vi "Main 手動測試.vi"() -> ()   [LabVIEW 2015]
uses:
  <vilib>/Utility/miscctls.llb/LVPointTypeDef.ctl
  2.0_Function/Function_VISA/Control/Control_Motion Action.ctl
  2.0_Function/Function_VISA/Control/Control_Axis Number.ctl
  <vilib>/Instr/_visa.llb/Select Event Type.ctl
panel:
  out "急停":bool
  out "DI":bool[][](array[boolean])
  in  "Time":u32=15000
  in  "儲存日檢位":path=path "D:/全域高斯機 參數/Daily Check"
  in  "儲存每日檢測位":bool
  out "量測值(T)":dbl format="%.1f"
  in  "單步角度(degree)":dbl=1.0 format="%#_13g"
  in  "確認離開":bool
  in  "單步距離(mm)":dbl=1.0 format="%#_13g"
  in  "-Rotation":bool
  in  "匯入硬體參數":path=path "D:/全域高斯機 參數/Paremeter"
  in  "目前位置":T1
  in  "軸參數":T2={"Name"="7", "VISA In"="COM2", "R"=0.0, "Y"=0.0, "Z"=0.0, "θ"=0.0, "最大值"=2.0, "最小值"=0.0, "VISA Data"={"Baud rate"=115200, "Data bits"=8, "Parity"=enum."Even", "Stop bits"=10, "Flow control"=0}, "Paremeter"={"Scan speed"=4, "Power"=2, "Angle"=0.0, "X"=3000, "X"=30000, "Xc"=30000}, "DAQ Paremeter"={"Task In"="CalibrationTest", "Physical Channels"="Dev1/ai0", "Max Value"=10.0, "Min Value"=-10.0, "Rate"=5.0}} {"DAQ Paremeter"."Rate" format="%0.2f"; "DAQ Paremeter"."Min Value" format="%0.2f"; "DAQ Paremeter"."Max Value" format="%0.2f"; "VISA Data"."Stop bits" items=["1.0"=10, "1.5"=15, "2.0"=20]; "VISA Data"."Flow control" items=["None", "XON/XOFF", "RTS/CTS", "XON/XOFF & RTS/CTS", "DTR/DSR", "XON/XOFF & DTR/DSR"]; "VISA Data"."Data bits" min=5 max=8 step=1; "Paremeter"."Power" items=["Abs"=2, "Rel"=3]; "Paremeter"."Scan speed" items=["X"=1, "Y"=2, "Z"=3, "Rotation"=4]}
  out "手動測試-Action":T5
  in  "+Z":bool
  in  "-Z":bool
  in  "All Home":bool
  in  "All Servo ON/off":bool
  in  "Rotation":bool
  in  "+X":bool
  in  "-X":bool
  in  "-Y":bool
  in  "+Y":bool
  in  "離開":bool
  # "手動測試"
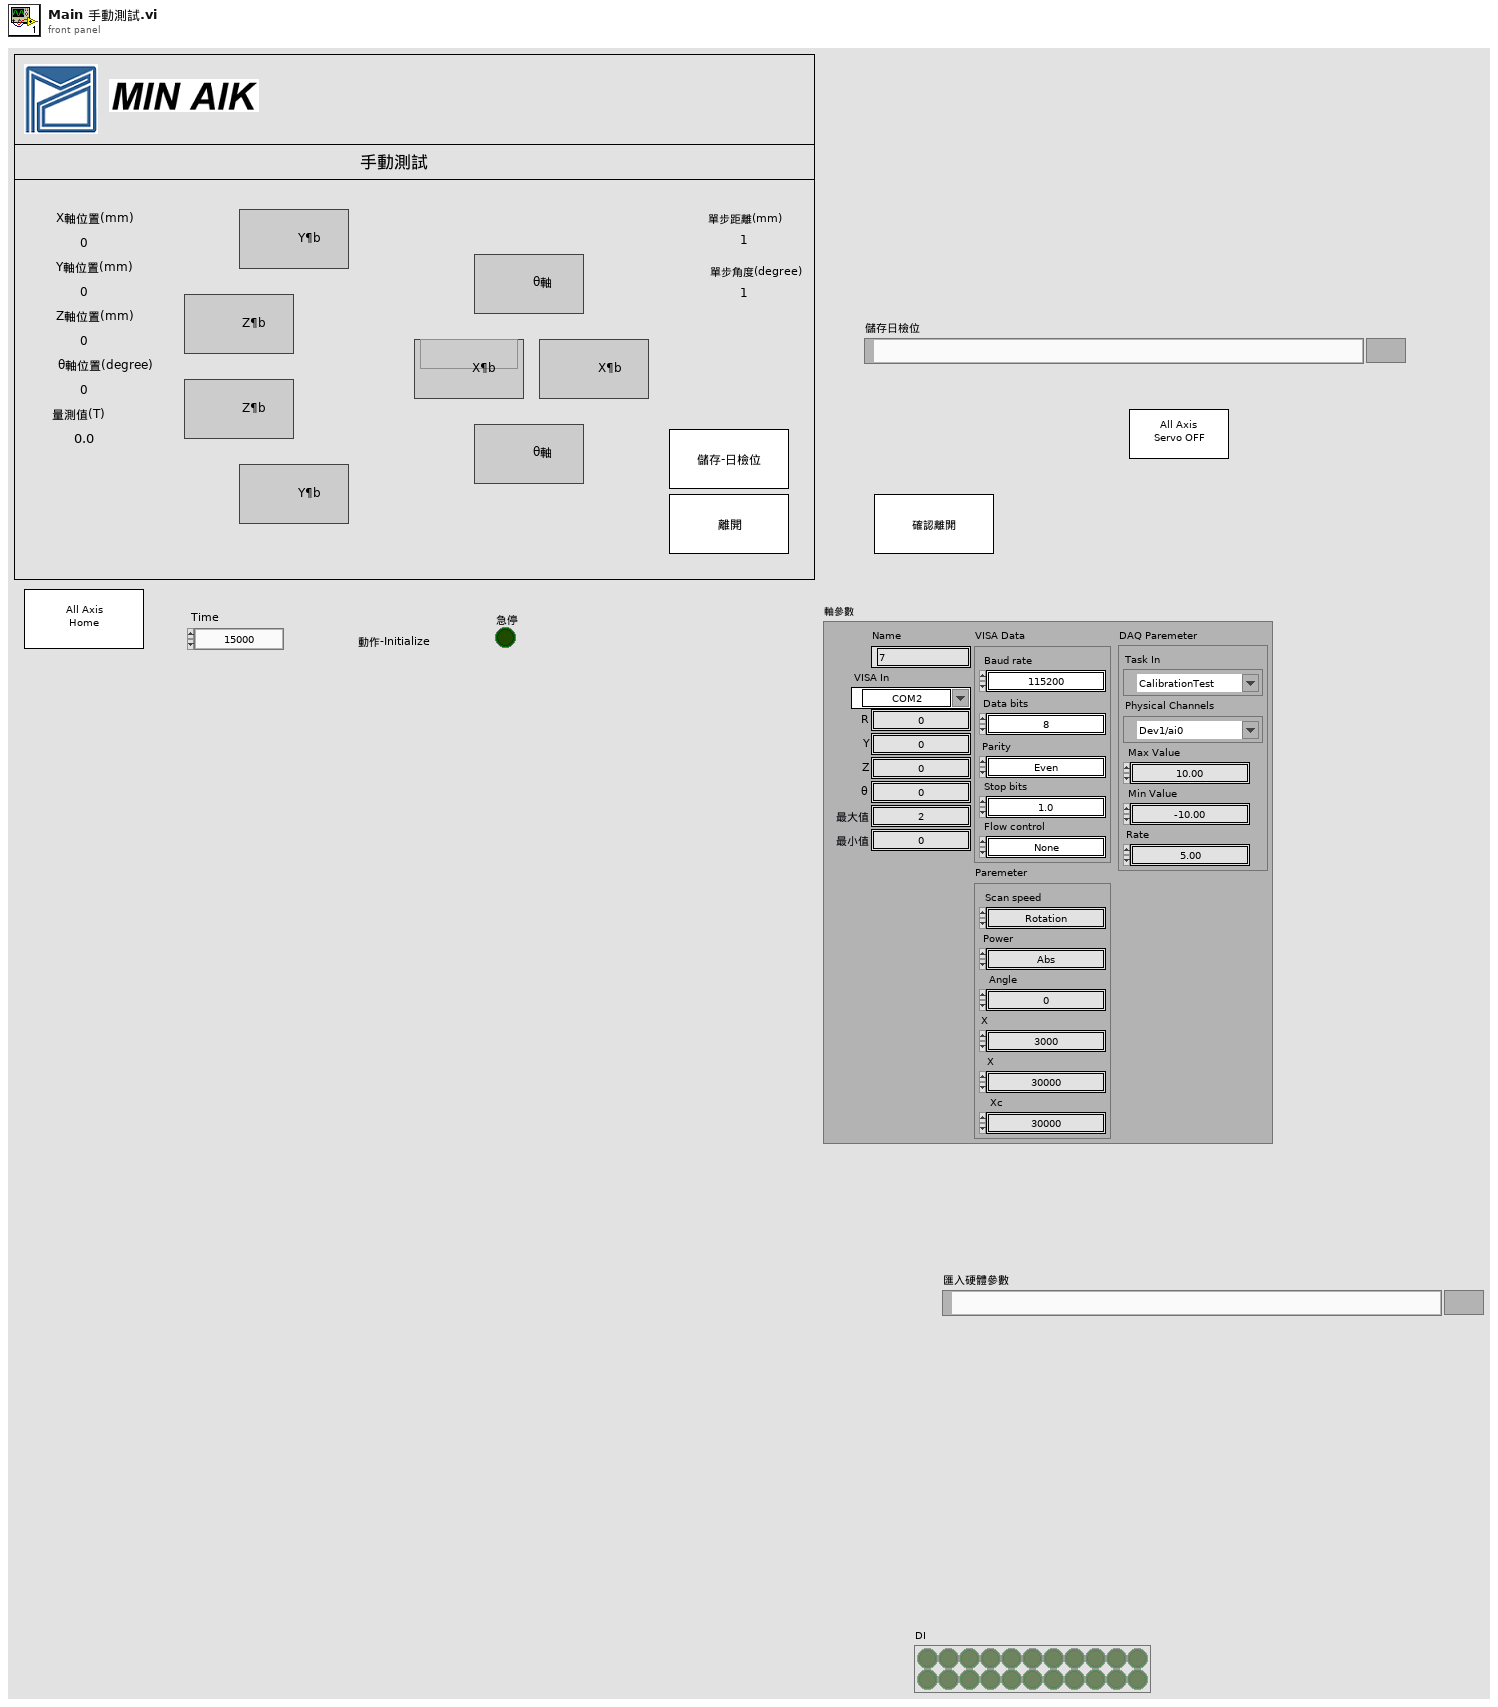
[diagram p1: front panel]
types:
  T1 = cluster{"X軸位置(mm)":dbl, "Y軸位置(mm)":dbl, "Z軸位置(mm)":dbl, "θ軸位置(degree)":dbl}
  T2 = typedef "Control_軸參數.ctl" = cluster{"Name":string, "VISA In":refnum<visa-resource-name>, "R":dbl, "Y":dbl, "Z":dbl, "θ":dbl, "最大值":dbl, "最小值":dbl, "VISA Data":cluster{"Baud rate":u32, "Data bits":u16, "Parity":enum16{"None", "Odd", "Even", "Mark", "Space"}, "Stop bits":u16, "Flow control":u16}, "Paremeter":T3, "DAQ Paremeter":cluster{"Task In":refnum<k21>, "Physical Channels":tag, "Max Value":dbl, "Min Value":dbl, "Rate":dbl}}
  T3 = typedef "Control_手動測試_軸參數.ctl" = cluster{"Scan speed":T4, "Power":u16, "Angle":dbl, "X":i32, "X":i32, "Xc":i32}
  T4 = typedef "Control_Axis Number.ctl" = u16
  T5 = typedef "Control_手動測試_手動測試 Action.ctl" = enum16{"動作-Initialize", "動作-All Axis Sarvo", "動作-All Axis Home", "動作-Exit", "動作-X移動+", "動作-X移動-", "動作-Y移動+", "動作-Y移動-", "動作-Z移動+", "動作-Z移動-", "動作-θ移動+", "動作-θ移動-", "1.0 ¶b-ªì©l¤Æ", "    1.1 ¶b-¶×¤J°Ñ¼Æ", "2.0 ¶b-X¦^­ìÂI", "    2.1 ¶b-Xª¬ºA", "    2.2 ¶b-X²¾°Ê", "    2.3 ¶b-X²¾°Êª¬ºA", "    2.4 ¶b-X¦ì¸m", "    2.5 ¶b-X¶×¤J°Ñ¼Æ", "3.0 ¶b-Y¦^­ìÂI", "    3.1 ¶b-Yª¬ºA", "    3.2 ¶b-Y²¾°Ê", "    3.3 ¶b-Y²¾°Êª¬ºA", "    3.4 ¶b-Y¦ì¸m", "    3.5 ¶b-Y¶×¤J°Ñ¼Æ", "4.0 ¶b-Z¦^­ìÂI", "    4.1 ¶b-Zª¬ºA", "    4.2 ¶b-Z²¾°Ê", "    4.3 ¶b-Z²¾°Êª¬ºA", "    4.4 ¶b-Z¦ì¸m", "    4.5 ¶b-Z¶×¤J°Ñ¼Æ", "5.0 ¶b-£c¦^­ìÂI", "    5.1 ¶b-£cª¬ºA", "    5.2 ¶b-£c²¾°Ê", "    5.3 ¶b-£c²¾°Êª¬ºA", "    5.4 ¶b-£c¦ì¸m", "    5.5 ¶b-£c¶×¤J°Ñ¼Æ", "6.0 ¶b-µ¥«Ý", "7.0 ¶b-µ²§ô", "8.0 量測", "    8.1 量測-初始化", "    8.2 量測-量測", "    8.2 量測-顯示結果", "    8.3 量測-離開", "9.0 等待", "10.0 離開", "    10.1 離開程式", "11.0 錯誤", "    11.1 錯誤-顯示錯誤", "    11.2 錯誤-急停"}
  T6 = typedef "Control_Measure_VISA action.ctl" = enum16{"1.0 Initialize", "2.0 Power ON", "2.1 Prower OFF", "2.2 Real", "2.3 Hold", "2.4 Reset", "2.5 DC Mode", "2.5.2 DC*10 Mode", "2.5.3 AC*10 Mode", "2.6 Write Commend", "2.7 Write Commend(Power)", "3.0 Read State", "3.1 Read Value", "4.0 Clear", "5.0 Close", "6.0 Idle"}
  T7 = typedef "Select Event Type.ctl" = u32
  T8 = typedef "LVPointTypeDef.ctl" = cluster{"Horizontal":i16, "Vertical":i16}
  T9 = typedef "Control_每日點檢_位置.ctl" = cluster{"目前位置":cluster{"X (mm)":dbl, "Y (mm)":dbl, "Z (mm)":dbl, "θ (degree)":dbl}, "Value(T)":dbl}
  T10 = typedef "Control_Main_Trigger Action Out.ctl" = enum16{"Hold", "Stop", "Start"}
  T11 = typedef "Control_Motion Action.ctl" = enum16{"Servo On", "Servo Off", "Homing", "Set Position", "Set Speed", "Set Acc", "Set Deacc", "Start Move", "Read Status", "Read Position"}
  T12 = enum16{"Open Connect", "Write and Read", "Close Connect"}
  T13 = cluster{"Baud rate":u32, "Data bits":u16, "Parity":enum16{"None", "Odd", "Even", "Mark", "Space"}, "Stop bits":u16, "Flow control":u16}
  T14 = cluster{"M0_R":bool, "M1_R":bool, "M2_R":bool, "M3_R":bool, "M4_R":bool, "M5_R":bool, "WNG":bool, "ALM":bool, "Strart_R":bool, "Step_Out":bool, "Move":bool, "Home_P":bool, "FreeUse1":bool, "Ready":bool, "FreeUse2":bool, "AREA":bool}
  T15 = typedef "Control_Bounce Window_Main_FGV_Error Action.ctl" = enum16{"Try Again", "Stop"}
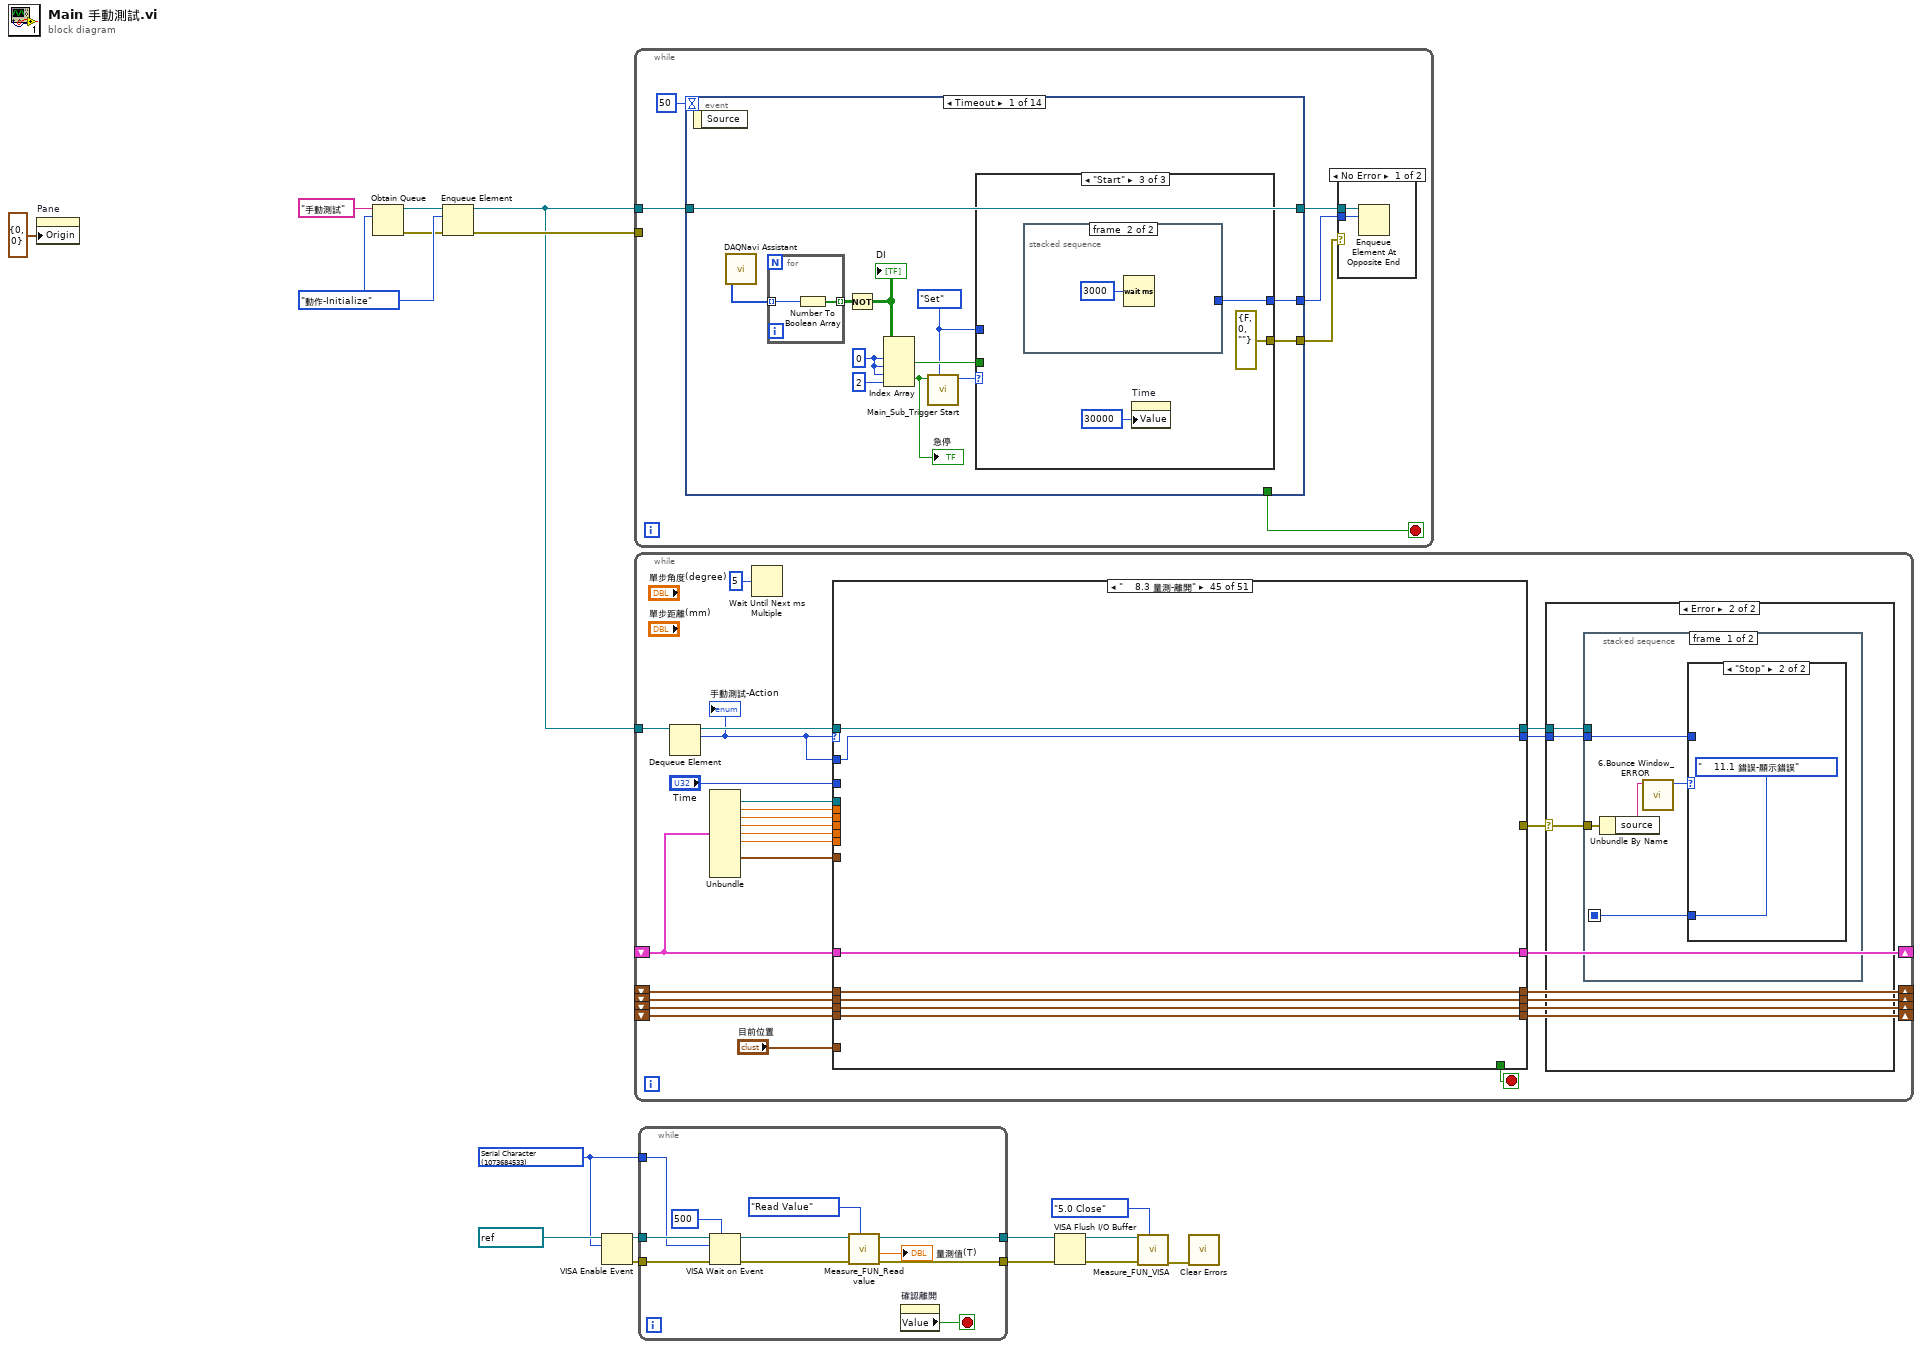
[diagram p0: block diagram]
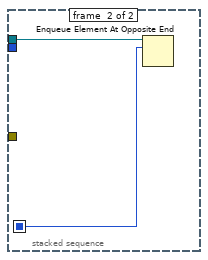
[diagram p4: hidden frame]
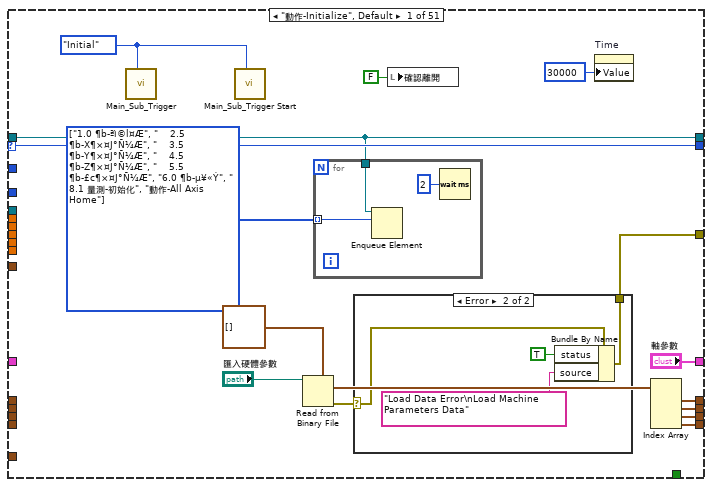
[diagram p5: hidden frame]
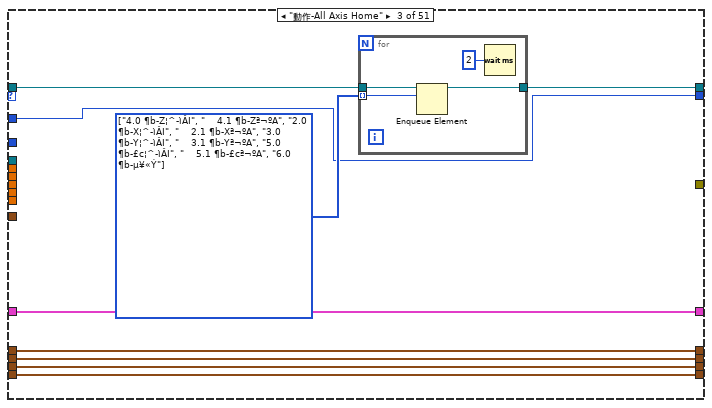
[diagram p8: hidden frame]
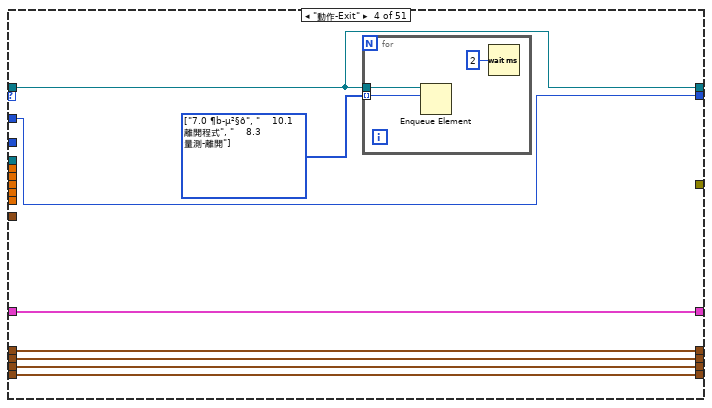
[diagram p9: hidden frame]
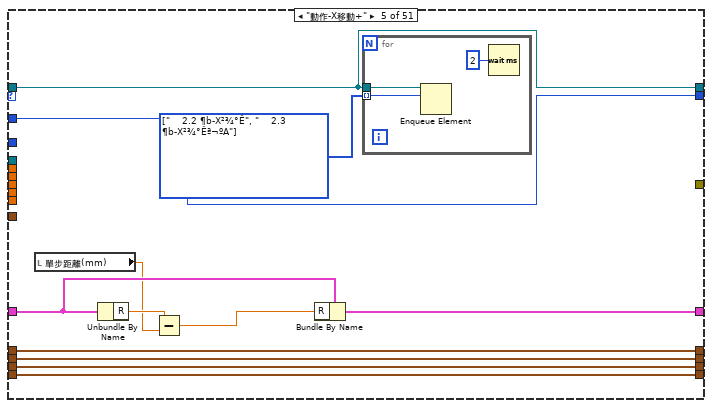
[diagram p10: hidden frame]
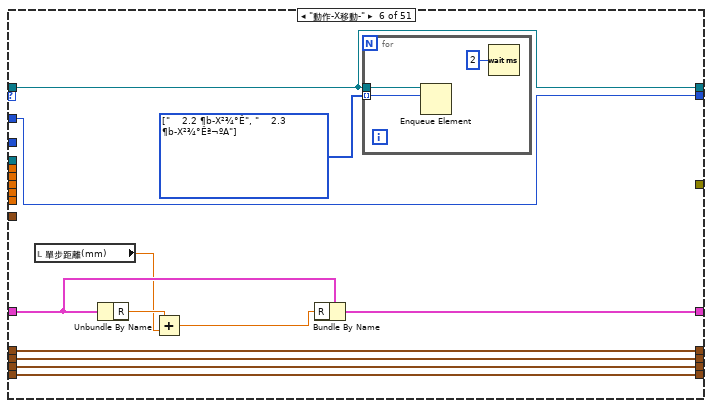
[diagram p11: hidden frame]
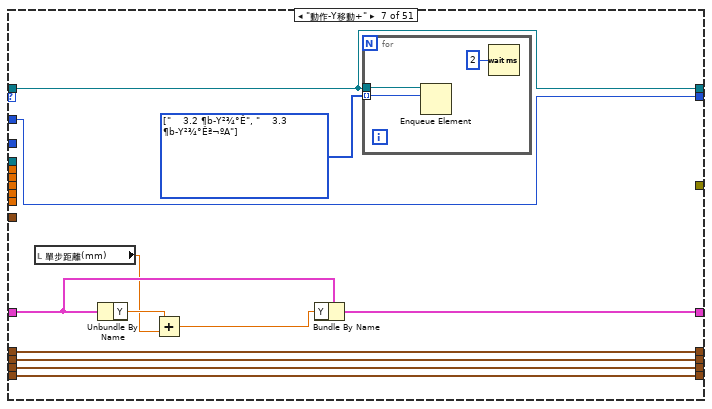
[diagram p12: hidden frame]
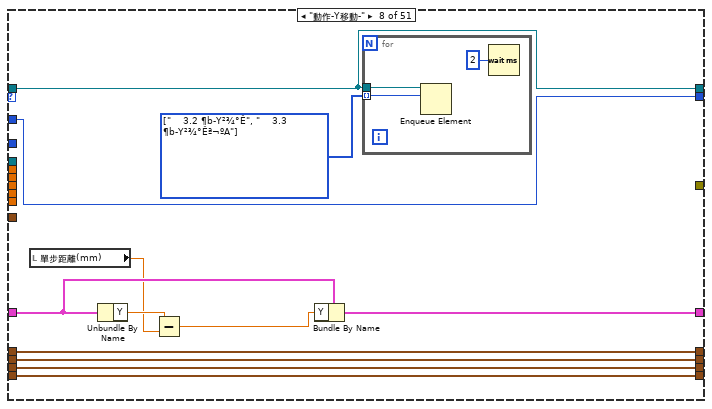
[diagram p13: hidden frame]
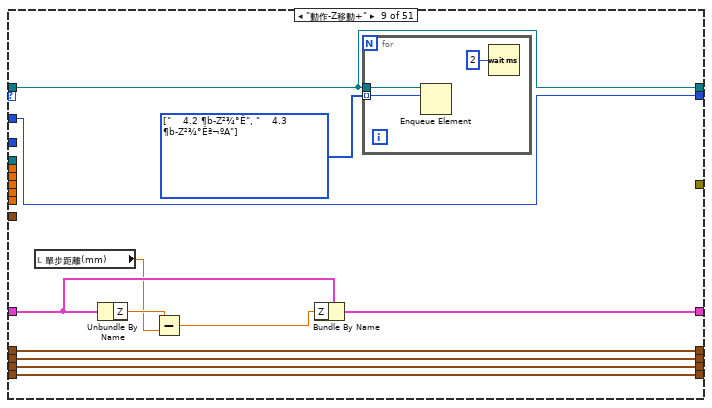
[diagram p14: hidden frame]
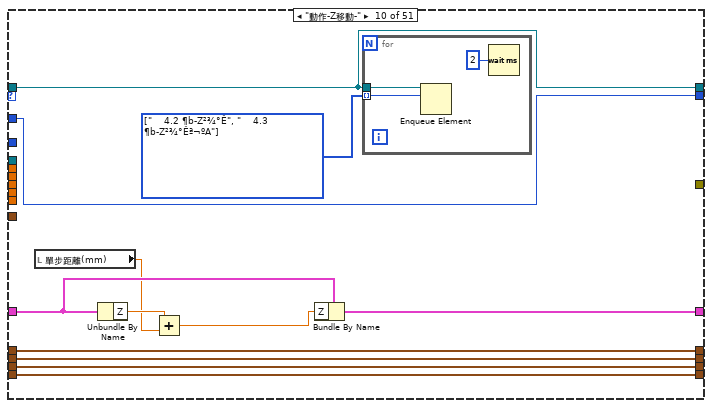
[diagram p15: hidden frame]
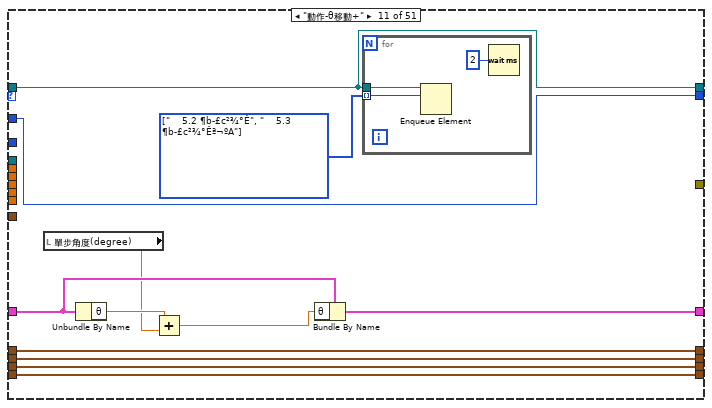
[diagram p16: hidden frame]
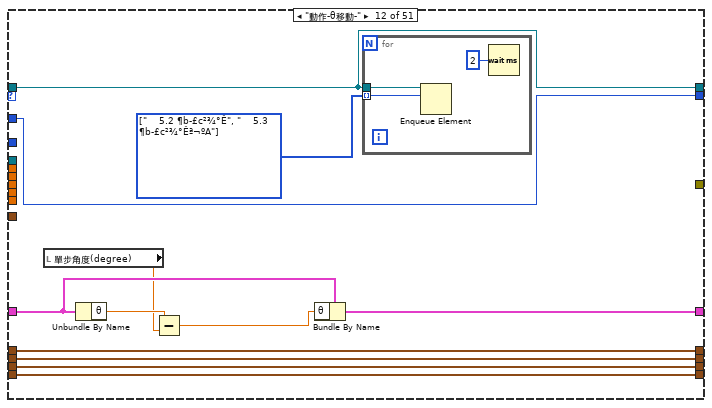
[diagram p17: hidden frame]
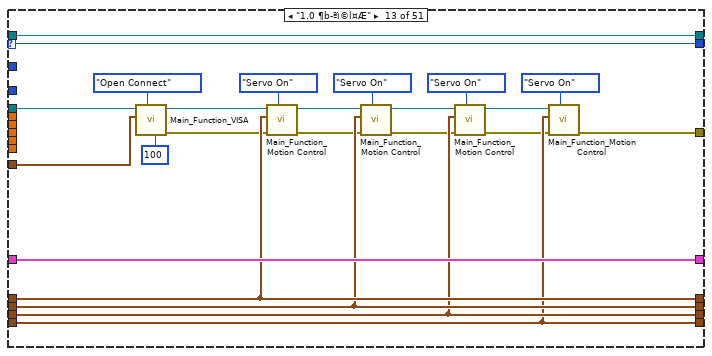
[diagram p18: hidden frame]
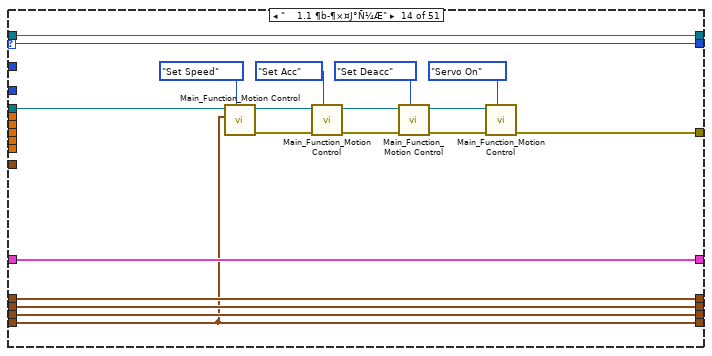
[diagram p19: hidden frame]
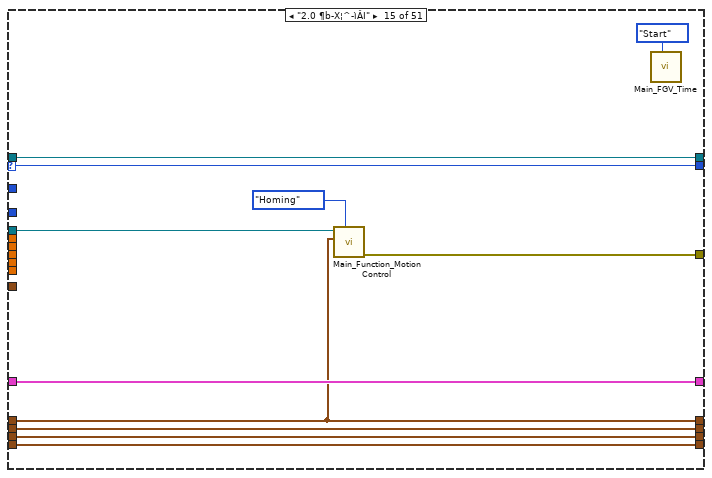
[diagram p20: hidden frame]
diagram:
  w5 = T7 1073684533 items=["Service Request"=1073684491, "Trigger"=3221168138, "Clear"=1073684493, "VXI Signal"=1073684512, "VXI/VME Interrupt"=3221168161, "VXI/VME Sysfail"=1073684509, "VXI/VME Sysreset"=1073684510, "GPIB CIC"=1073684498, "GPIB Talk"=1073684499, "GPIB Listen"=1073684500, "PXI Interrupt"=1073684514, "Serial Break"=1073684515, "Serial TermChar"=1073684516, "Serial CTS"=1073684521, "Serial DSR"=1073684522, "Serial DCD"=1073684524, "Serial RI"=1073684526, "Serial Character"=1073684533, "USB Interrupt"=1073684535, "All Enabled"=1073709055] ("Event Type")
  w14 = Control_手動測試_手動測試_Action."動作-Initialize" ("手動測試-Action")
  n1 = property on="Pane" class="Pane"("Origin"=T8 {"Horizontal"=0, "Vertical"=0}) -> ()  [unwired: 2 in, 2 out]
  n2 = Obtain Queue(name (unnamed)="手動測試", element data type=w14) -> (queue out=w15:refnum<queue>, error out=w13:errorcluster)  [unwired: 3 in, 1 out]
  n3 = Enqueue Element(queue=w15, element=w14, error in (no error)=w13) -> (queue out=w11:refnum<queue>, error out=w12:errorcluster)  [unwired: 1 in, 1 out]
  n4 = VISA Enable Event(10:w5, 11:refnum<visa-resource-name> "COM9" ("VISA resource name")) -> (0:w6:errorcluster, 3:w7:refnum<visa-resource-name>)  [unwired: 2 in]
  n5 = while {
    tunnel: w12 -> [_]
    tunnel: w11 -> [w23]
    stop <- w20 stop-if-true
    n6 = event shown="[0] Timeout" {
      selector: _ -> [_ _ _ _ _ _ _ _ _ _ _ _ _ _]
      dyn-events: _ -> [_ _ _ _ _ _ _ _ _ _ _ _ _ _]
      timeout: 50 -> [_ _ _ _ _ _ _ _ _ _ _ _ _ _]
      tunnel: w23 -> [w26 w61 w63 w71 w73 w76 w78 w80 w82 w84 w86 w88 w90 w92]
      tunnel: [w26 w61 w63 w71 w73 w76 w78 w80 w82 w84 w86 w88 w90 w92] -> w22
      tunnel: [w27 Control_手動測試_手動測試_Action."動作-All Axis Sarvo" ("手動測試-Action") Control_手動測試_手動測試_Action."動作-All Axis Home" ("手動測試-Action") _ Control_手動測試_手動測試_Action."動作-Exit" ("手動測試-Action") _ Control_手動測試_手動測試_Action."動作-X移動+" ("手動測試-Action") Control_手動測試_手動測試_Action."動作-X移動-" ("手動測試-Action") Control_手動測試_手動測試_Action."動作-Y移動+" ("手動測試-Action") Control_手動測試_手動測試_Action."動作-Y移動-" ("手動測試-Action") Control_手動測試_手動測試_Action."動作-Z移動+" ("手動測試-Action") Control_手動測試_手動測試_Action."動作-Z移動-" ("手動測試-Action") Control_手動測試_手動測試_Action."動作-θ移動+" ("手動測試-Action") Control_手動測試_手動測試_Action."動作-θ移動-" ("手動測試-Action")] -> w21
      tunnel: [_ _ _ _ _ TRUE _ _ _ _ _ _ _ _] -> w20
      tunnel: [w28 _ _ errorcluster {"status"=TRUE, "code"=0, "source"=""} ("error in (no error)") _ errorcluster {"status"=TRUE, "code"=0, "source"=""} ("error in (no error)") _ _ _ _ _ _ _ _] -> w19
      event Timeout {
        w29 = enum16{"Initial", "Set"}."Set" ("Trigger_Action")
        w34 = 0 ("index (row)")
        n7 = event-data() -> ()  [unwired: 1 in, 1 out]
        n8 = call "DAQNavi Assistant"() -> ("dataOut(U8Array)"=w37:u8[])  [unwired: 26 in, 1 out]
        n9 = for {
          tunnel: w37 -> [w59] mode=indexing
          tunnel: [w58] -> w36 mode=indexing
          n10 = Number To Boolean Array(number=w59) -> (Boolean array=w58:bool[])
        }
        n11 = Not(x=w36) -> (.not. x?=w35:bool[][])
        "DI" <- w35
        n12 = Index Array(array=w35, index (row) #1=w34, index (col) #1=w34, index (row) #2=w34, index (col) #2=2 ("disabled index (col)")) -> (element #1=w30:bool, element #2=w32:bool)
        "急停" <- w32
        n13 = call "Main_Sub_Trigger Start.vi"("Trigger_Action"=w29, "Trigger"=w32) -> ("Trigger_Action Out"=w31:T10)  [unwired: 9 in]
        n14 = case shown="\"Start\"" w31 {
          tunnel: w30 -> [w40 _ _]
          tunnel: w29 -> [_ _ _]
          tunnel: [w42 errorcluster {"status"=FALSE, "code"=0, "source"=""} ("Error Out") errorcluster {"status"=FALSE, "code"=0, "source"=""} ("Error Out")] -> w28
          tunnel: [w38 Control_手動測試_手動測試_Action."    11.2 錯誤-急停" ("手動測試-Action 2") w54] -> w27
          frame "Hold", Default {
            n15 = call "Main_Sub_Trigger.vi"("Trigger_Action"=enum16{"Initial", "Set"}."Set", "Trigger"=w40) -> ("Trigger_Action Out"=w39:T10)  [unwired: 9 in]
            n16 = case shown="\"Start\"" w39 {
              tunnel: [errorcluster {"status"=TRUE, "code"=0, "source"=""} ("Error Out") errorcluster {"status"=FALSE, "code"=0, "source"=""} ("Error Out") errorcluster {"status"=FALSE, "code"=0, "source"=""} ("Error Out")] -> w42
              tunnel: [Control_手動測試_手動測試_Action."9.0 等待" ("手動測試-Action") Control_手動測試_手動測試_Action."9.0 等待" ("手動測試-Action") Control_手動測試_手動測試_Action."9.0 等待" ("手動測試-Action")] -> w38
              frame "Hold", Default {
              }
              frame "Stop" {
              }
              frame "Start" {
              }
            }
          }
          frame "Stop" {
            n17 = property on="Time" class="DigNum (strict)"("Value"=u32 0 ("Time")) -> ()  [unwired: 2 in, 2 out]
            n18 = call "5.Bounce Window_MSG.vi"("MSG In"="急停！") -> ()  [unwired: 11 in]
          }
          frame "Start" {
            n19 = stacked-sequence {
              tunnel: [Control_手動測試_手動測試_Action."動作-Initialize" ("手動測試-Action 2") _] -> w54
              frame #0 {
              }
              frame #1 {
                n20 = Wait (ms)(milliseconds to wait=u32 3000) -> ()  [unwired: 1 out]
              }
            }
            n21 = property on="Time" class="DigNum (strict)"("Value"=u32 30000 ("Time")) -> ()  [unwired: 2 in, 2 out]
          }
        }
      }
      event "All Servo ON/off": Value Change {
        n22 = event-data() -> ()  [unwired: 1 in, 1 out]
      }
      event "All Home": Value Change {
        n23 = event-data() -> ()  [unwired: 1 in, 1 out]
      }
      event "儲存每日檢測位": Value Change {
        n24 = event-data() -> ()  [unwired: 1 in, 1 out]
        n25 = local read "量測值(T)"() -> (w67:dbl)
        n26 = local read "目前位置"() -> (w68:T1)
        n27 = Bundle By Name(cluster=T9 {"目前位置"={"X (mm)"=0.0, "Y (mm)"=0.0, "Z (mm)"=0.0, "θ (degree)"=0.0}, "Value(T)"=1174.5} ("Daily Chack"), "目前位置"=w68, "Value(T)"=w67) -> (w66:T9)
        n28 = Write to Binary File(file (use dialog)="儲存日檢位", data=w66) -> (error out=w64:errorcluster)  [unwired: 4 in, 2 out]
        n29 = call <vilib>:"Clear Errors.vi"("error in (no error)"=w64) -> ()  [unwired: 5 in, 2 out]
      }
      event "離開": Value Change {
        n30 = event-data() -> ()  [unwired: 1 in, 1 out]
      }
      event "確認離開": Value Change {
        n31 = event-data() -> ()  [unwired: 1 in, 1 out]
      }
      event "+X": Value Change {
        n32 = event-data() -> ()  [unwired: 1 in, 1 out]
      }
      event "-X": Value Change {
        n33 = event-data() -> ()  [unwired: 1 in, 1 out]
      }
      event "+Y": Value Change {
        n34 = event-data() -> ()  [unwired: 1 in, 1 out]
      }
      event "-Y": Value Change {
        n35 = event-data() -> ()  [unwired: 1 in, 1 out]
      }
      event "+Z": Value Change {
        n36 = event-data() -> ()  [unwired: 1 in, 1 out]
      }
      event "-Z": Value Change {
        n37 = event-data() -> ()  [unwired: 1 in, 1 out]
      }
      event "Rotation": Value Change {
        n38 = event-data() -> ()  [unwired: 1 in, 1 out]
      }
      event "-Rotation": Value Change {
        n39 = event-data() -> ()  [unwired: 1 in, 1 out]
      }
    }
    n40 = case shown="No Error" w19 {
      tunnel: w22 -> [w25 _]
      tunnel: w21 -> [w24 _]
      frame No Error {
        n41 = Enqueue Element At Opposite End(queue=w25, element=w24) -> ()  [unwired: 2 in, 3 out]
      }
      frame Error {
      }
    }
  }
  n42 = while {
    tunnel: w11 -> [w119]
    shift-right: [w109] -> _
    shift-left: _ -> [w99]
    shift-right: [w108] -> _
    shift-left: _ -> [w104]
    shift-right: [w107] -> _
    shift-left: _ -> [w103]
    shift-right: [w106] -> _
    shift-left: _ -> [w102]
    shift-right: [w105] -> _
    shift-left: _ -> [w101]
    stop <- w111 stop-if-true
    n43 = Dequeue Element(queue=w119) -> (queue out=w94:refnum<queue>, element=w93:T5)  [unwired: 2 in, 2 out]
    "手動測試-Action" <- w93
    n44 = Unbundle(w99) -> ("VISA In"=w113:refnum<visa-resource-name>, "R"=w118:dbl, "Y"=w117:dbl, "Z"=w116:dbl, "θ"=w115:dbl, "最大值"=w114:dbl, "VISA Data"=w100:T13)  [unwired: 4 out]
    n45 = Wait Until Next ms Multiple(millisecond multiple=u32 5 ("milliseconds to wait")) -> ()  [unwired: 1 out]
    n46 = case shown="\"    8.3 量測-離開\"" w93 {
      selector: w93 -> [w135 w156 _ _ _ _ _ _ _ _ _ _ w321 w331 w351 w361 _ _ _ _ _ w532 _ w600 _ _ _ _ w746 _ _ _ _ _ _ _ _ _ _ _ _ w1065 _ _ _ w1106 _ _ w1133 _ _]
      tunnel: w94 -> [w134 w157 w171 w182 w197 w210 w223 w240 w255 w270 w285 w300 w322 w332 w352 w372 w412 w434 w478 w500 w520 w535 w580 w601 w647 w669 w689 w701 w748 w767 w814 w836 w856 w866 w916 w936 w983 w1005 w1024 w1036 w1059 w1066 w1086 w1093 w1100 w1107 w1114 w1121 w1134 w1143 w1151]
      tunnel: w118 -> [_ _ _ _ _ _ _ _ _ _ _ _ _ _ _ _ w419 _ _ _ _ _ _ _ _ _ _ _ _ _ _ _ _ _ _ _ _ _ _ _ _ _ _ _ _ _ _ _ _ _ _]
      tunnel: w117 -> [_ _ _ _ _ _ _ _ _ _ _ _ _ _ _ _ _ _ _ _ _ _ w587 _ _ _ _ _ _ _ _ _ _ _ _ _ _ _ _ _ _ _ _ _ _ _ _ _ _ _ _]
      tunnel: w116 -> [_ _ _ _ _ _ _ _ _ _ _ _ _ _ _ _ _ _ _ _ _ _ _ _ _ _ _ _ w755 _ _ _ _ _ _ _ _ _ _ _ _ _ _ _ _ _ _ _ _ _ _]
      tunnel: w115 -> [_ _ _ _ _ _ _ _ _ _ _ _ _ _ _ _ _ _ _ _ _ _ _ _ _ _ _ _ _ _ _ _ _ _ w923 _ _ _ _ _ _ _ _ _ _ _ _ _ _ _ _]
      tunnel: w114 -> [_ _ _ _ _ _ _ _ _ _ _ _ _ _ _ _ _ _ _ _ _ _ _ _ _ _ _ _ _ _ _ _ _ _ _ _ _ _ _ _ _ _ _ _ _ _ _ _ _ _ _]
      tunnel: w113 -> [_ _ _ _ _ _ _ _ _ _ _ _ w330 w335 w359 w371 w420 w440 w486 w506 w527 w541 w588 w609 w656 w671 w696 w709 w756 w776 w822 w839 w863 w876 w924 w944 w991 w1008 w1031 w1043 _ _ _ _ _ _ _ _ _ _ _]
      tunnel: "目前位置" -> [_ _ _ _ _ _ _ _ _ _ _ _ _ _ _ _ _ _ w485 _ _ _ _ _ w655 _ _ _ _ _ w821 _ _ _ _ _ w990 _ _ _ _ _ _ _ _ _ _ _ _ _ _]
      tunnel: [_ _ _ _ _ _ _ _ _ _ _ _ _ _ _ _ _ _ _ _ _ _ _ _ _ _ _ _ _ _ _ _ _ _ _ _ _ _ _ _ _ _ _ _ _ _ _ TRUE _ _ _] -> w111
      tunnel: ["軸參數" w162 w169 w181 w194 w208 w224 w238 w253 w268 w283 w298 w329 w349 w358 w370 w418 w439 w484 w517 w526 w540 w586 w608 w654 w676 w695 w708 w750 w775 w820 w853 w862 w875 w922 w943 w989 w1019 w1030 w1042 w1060 w1080 w1087 w1094 w1101 w1108 w1119 w1127 w1135 w1141 w1149] -> w109
      tunnel: w99 -> [_ w162 w169 w181 w193 w209 w225 w239 w254 w269 w284 w299 w329 w349 w358 w370 w418 w439 w484 w517 w526 w540 w586 w608 w654 w676 w695 w708 w750 w775 w820 w853 w862 w875 w922 w943 w989 w1019 w1030 w1042 w1060 w1080 w1087 w1094 w1101 w1108 w1119 w1127 w1135 w1141 w1149]
      tunnel: [w143 w161 w168 w180 w192 w207 w222 w237 w252 w267 w282 w297 w328 w348 w354 w366 w414 w435 w480 w505 w525 w539 w585 w607 w652 w675 w694 w707 w754 w774 w819 w852 w861 w874 w921 w942 w988 w1022 w1029 w1040 w1064 w1084 w1091 w1098 w1105 w1112 w1118 w1126 w1132 w1140 w1148] -> w108
      tunnel: [w142 w160 w167 w179 w191 w206 w221 w236 w251 w266 w281 w296 w327 w347 w357 w369 w417 w438 w483 w516 w522 w536 w582 w604 w649 w672 w693 w706 w753 w773 w818 w851 w860 w873 w920 w941 w987 w1021 w1028 w1039 w1063 w1083 w1090 w1097 w1104 w1111 w1117 w1125 w1131 w1139 w1147] -> w107
      tunnel: [w141 w159 w166 w178 w190 w205 w220 w235 w250 w265 w280 w295 w326 w346 w356 w368 w416 w437 w482 w515 w524 w538 w584 w606 w651 w674 w691 w704 w751 w771 w816 w838 w859 w872 w919 w940 w986 w1007 w1027 w1038 w1062 w1082 w1089 w1096 w1103 w1110 w1116 w1124 w1130 w1138 w1146] -> w106
      tunnel: [w140 w158 w165 w177 w189 w204 w219 w234 w249 w264 w279 w294 w325 w334 w355 w367 w415 w436 w481 w514 w523 w537 w583 w605 w650 w673 w692 w705 w752 w772 w817 w850 w858 w871 w918 w939 w985 w1020 w1026 w1037 w1061 w1081 w1088 w1095 w1102 w1109 w1115 w1123 w1129 w1137 w1145] -> w105
      tunnel: w104 -> [_ w161 w168 w180 w192 w207 w222 w237 w252 w267 w282 w297 w328 w348 w354 w366 w414 w435 w480 w505 w525 w539 w585 w607 w652 w675 w694 w707 w754 w774 w819 w852 w861 w874 w921 w942 w988 w1022 w1029 w1040 w1064 w1084 w1091 w1098 w1105 w1112 w1118 w1126 w1132 w1140 w1148]
      tunnel: w103 -> [_ w160 w167 w179 w191 w206 w221 w236 w251 w266 w281 w296 w327 w347 w357 w369 w417 w438 w483 w516 w522 w536 w582 w604 w649 w672 w693 w706 w753 w773 w818 w851 w860 w873 w920 w941 w987 w1021 w1028 w1039 w1063 w1083 w1090 w1097 w1104 w1111 w1117 w1125 w1131 w1139 w1147]
      tunnel: w102 -> [_ w159 w166 w178 w190 w205 w220 w235 w250 w265 w280 w295 w326 w346 w356 w368 w416 w437 w482 w515 w524 w538 w584 w606 w651 w674 w691 w704 w751 w771 w816 w838 w859 w872 w919 w940 w986 w1007 w1027 w1038 w1062 w1082 w1089 w1096 w1103 w1110 w1116 w1124 w1130 w1138 w1146]
      tunnel: w101 -> [_ w158 w165 w177 w189 w204 w219 w234 w249 w264 w279 w294 w325 w334 w355 w367 w415 w436 w481 w514 w523 w537 w583 w605 w650 w673 w692 w705 w752 w772 w817 w850 w858 w871 w918 w939 w985 w1020 w1026 w1037 w1061 w1081 w1088 w1095 w1102 w1109 w1115 w1123 w1129 w1137 w1145]
      tunnel: w100 -> [_ _ _ _ _ _ _ _ _ _ _ _ w324 _ _ _ _ _ _ _ _ _ _ _ _ _ _ _ _ _ _ _ _ _ _ _ _ _ _ w1041 _ _ _ _ _ _ _ _ _ _ _]
      tunnel: [w136 _ _ _ _ _ _ _ _ _ _ _ w323 w333 w353 w362 w413 w429 w479 w501 w521 w530 w581 w602 w648 w670 w690 w702 w749 w769 w815 w837 w857 w868 w917 w937 w984 w1006 w1025 w1034 _ w1067 _ _ _ _ _ _ _ _ _] -> w98
      tunnel: [w135 w156 w163 w176 w187 w202 w217 w232 w247 w262 w277 w292 w321 w331 w351 w363 w410 w431 w477 w499 w518 w531 w578 w599 w646 w668 w687 w698 w746 w768 w813 w835 w854 w867 w914 w935 w982 w1004 w1023 w1033 w1058 w1065 w1085 w1092 w1099 w1106 w1113 w1120 w1133 w1136 w1144] -> w97
      tunnel: [w134 w157 w164 w182 w197 w210 w223 w240 w255 w270 w285 w300 w322 w332 w352 w372 w412 w434 w478 w500 w520 w535 w580 w601 w647 w669 w689 w701 w748 w767 w814 w836 w856 w866 w916 w936 w983 w1005 w1024 w1036 w1059 w1066 w1086 w1093 w1100 w1107 w1114 w1121 w1134 w1142 w1150] -> w96
      tunnel: "Time" -> [_ _ _ _ _ _ _ _ _ _ _ _ _ _ _ w364 _ w432 _ _ _ w534 _ w598 _ _ _ w700 _ w765 _ _ _ w865 _ w934 _ _ _ _ _ _ _ _ _ _ _ _ _ _ _]
      tunnel: w93 -> [_ _ w163 w176 w187 w202 w217 w232 w247 w262 w277 w292 _ _ _ _ w410 _ w477 w499 w518 _ w578 _ w646 w668 w687 _ _ _ w813 w835 w854 _ w914 _ w982 w1004 w1023 w1033 w1058 _ w1085 w1092 w1099 _ w1113 w1120 _ w1136 w1144]
      frame "動作-Initialize", Default {
        w133 = enum16{"Initial", "Set"}."Initial" ("Trigger_Action")
        n47 = call "Main_Sub_Trigger.vi"("Trigger_Action"=w133) -> ()  [unwired: 10 in, 1 out]
        n48 = call "Main_Sub_Trigger Start.vi"("Trigger_Action"=w133) -> ()  [unwired: 10 in, 1 out]
        n49 = Read from Binary File(5:T3[] [] ("各軸參數"), 11:"匯入硬體參數") -> (0:w138:errorcluster, 2:w137:T3[])  [unwired: 4 in, 2 out]
        n50 = for {
          tunnel: T5[] [enum."1.0 ¶b-ªì©l¤Æ", enum."    2.5 ¶b-X¶×¤J°Ñ¼Æ", enum."    3.5 ¶b-Y¶×¤J°Ñ¼Æ", enum."    4.5 ¶b-Z¶×¤J°Ñ¼Æ", enum."    5.5 ¶b-£c¶×¤J°Ñ¼Æ", enum."6.0 ¶b-µ¥«Ý", enum."    8.1 量測-初始化", enum."動作-All Axis Home"] -> [w154] mode=indexing
          tunnel: w134 -> [w153]
          n51 = Enqueue Element(queue=w153, element=w154) -> ()  [unwired: 2 in, 3 out]
          n52 = Wait (ms)(milliseconds to wait=u32 2 ("millisecond multiple")) -> ()  [unwired: 1 out]
        }
        n53 = case shown="Error" w138 {
          selector: w138 -> [w148 w152]
          tunnel: [w148 w149] -> w136
          frame No Error {
          }
          frame Error {
            n54 = Bundle By Name(cluster=w152, "status"=TRUE, "source"="Load Data Error\nLoad Machine Parameters Data") -> (w149:errorcluster)
          }
        }
        n55 = local write "確認離開"(FALSE ("確認離開")) -> ()
        n56 = property on="Time" class="DigNum (strict)"("Value"=u32 30000 ("Time")) -> ()  [unwired: 2 in, 2 out]
        n57 = Index Array(array=w137) -> (element #1=w143:T3, element #2=w142:T3, element #3=w141:T3, element #4=w140:T3)  [unwired: 4 in]
      }
      frame "動作-All Axis Sarvo" {
      }
      frame "動作-All Axis Home" {
        n58 = for {
          tunnel: w171 -> [w174]
          tunnel: T5[] [enum."4.0 ¶b-Z¦^­ìÂI", enum."    4.1 ¶b-Zª¬ºA", enum."2.0 ¶b-X¦^­ìÂI", enum."    2.1 ¶b-Xª¬ºA", enum."3.0 ¶b-Y¦^­ìÂI", enum."    3.1 ¶b-Yª¬ºA", enum."5.0 ¶b-£c¦^­ìÂI", enum."    5.1 ¶b-£cª¬ºA", enum."6.0 ¶b-µ¥«Ý"] -> [w173] mode=indexing
          tunnel: [w172] -> w164
          n59 = Enqueue Element(queue=w174, element=w173) -> (queue out=w172:refnum<queue>)  [unwired: 2 in, 2 out]
          n60 = Wait (ms)(milliseconds to wait=u32 2 ("millisecond multiple")) -> ()  [unwired: 1 out]
        }
      }
      frame "動作-Exit" {
        n61 = for {
          tunnel: w182 -> [w185]
          tunnel: T5[] [enum."7.0 ¶b-µ²§ô", enum."    10.1 離開程式", enum."    8.3 量測-離開"] -> [w184] mode=indexing
          n62 = Enqueue Element(queue=w185, element=w184) -> ()  [unwired: 2 in, 3 out]
          n63 = Wait (ms)(milliseconds to wait=u32 2 ("millisecond multiple")) -> ()  [unwired: 1 out]
        }
      }
      frame "動作-X移動+" {
        n64 = local read "單步距離(mm)"() -> (w188:dbl)
        n65 = Unbundle By Name(w193) -> ("R"=w196:dbl)
        n66 = Subtract(x=w196, y=w188) -> (x-y=w195:dbl)
        n67 = Bundle By Name(cluster=w193, "R"=w195) -> (w194:T2)
        n68 = for {
          tunnel: w197 -> [w200]
          tunnel: T5[] [enum."    2.2 ¶b-X²¾°Ê", enum."    2.3 ¶b-X²¾°Êª¬ºA"] -> [w199] mode=indexing
          n69 = Enqueue Element(queue=w200, element=w199) -> ()  [unwired: 2 in, 3 out]
          n70 = Wait (ms)(milliseconds to wait=u32 2 ("millisecond multiple")) -> ()  [unwired: 1 out]
        }
      }
      frame "動作-X移動-" {
        n71 = local read "單步距離(mm)"() -> (w203:dbl)
        n72 = Unbundle By Name(w209) -> ("R"=w212:dbl)
        n73 = Add(x=w212, y=w203) -> (x+y=w211:dbl)
        n74 = Bundle By Name(cluster=w209, "R"=w211) -> (w208:T2)
        n75 = for {
          tunnel: w210 -> [w215]
          tunnel: T5[] [enum."    2.2 ¶b-X²¾°Ê", enum."    2.3 ¶b-X²¾°Êª¬ºA"] -> [w214] mode=indexing
          n76 = Enqueue Element(queue=w215, element=w214) -> ()  [unwired: 2 in, 3 out]
          n77 = Wait (ms)(milliseconds to wait=u32 2 ("millisecond multiple")) -> ()  [unwired: 1 out]
        }
      }
      frame "動作-Y移動+" {
        n78 = local read "單步距離(mm)"() -> (w218:dbl)
        n79 = Unbundle By Name(w225) -> ("Y"=w227:dbl)
        n80 = Add(x=w227, y=w218) -> (x+y=w226:dbl)
        n81 = Bundle By Name(cluster=w225, "Y"=w226) -> (w224:T2)
        n82 = for {
          tunnel: w223 -> [w230]
          tunnel: T5[] [enum."    3.2 ¶b-Y²¾°Ê", enum."    3.3 ¶b-Y²¾°Êª¬ºA"] -> [w229] mode=indexing
          n83 = Enqueue Element(queue=w230, element=w229) -> ()  [unwired: 2 in, 3 out]
          n84 = Wait (ms)(milliseconds to wait=u32 2 ("millisecond multiple")) -> ()  [unwired: 1 out]
        }
      }
      frame "動作-Y移動-" {
        n85 = local read "單步距離(mm)"() -> (w233:dbl)
        n86 = Unbundle By Name(w239) -> ("Y"=w242:dbl)
        n87 = Subtract(x=w242, y=w233) -> (x-y=w241:dbl)
        n88 = Bundle By Name(cluster=w239, "Y"=w241) -> (w238:T2)
        n89 = for {
          tunnel: w240 -> [w245]
          tunnel: T5[] [enum."    3.2 ¶b-Y²¾°Ê", enum."    3.3 ¶b-Y²¾°Êª¬ºA"] -> [w244] mode=indexing
          n90 = Enqueue Element(queue=w245, element=w244) -> ()  [unwired: 2 in, 3 out]
          n91 = Wait (ms)(milliseconds to wait=u32 2 ("millisecond multiple")) -> ()  [unwired: 1 out]
        }
      }
      frame "動作-Z移動+" {
        n92 = local read "單步距離(mm)"() -> (w248:dbl)
        n93 = Unbundle By Name(w254) -> ("Z"=w257:dbl)
        n94 = Subtract(x=w257, y=w248) -> (x-y=w256:dbl)
        n95 = Bundle By Name(cluster=w254, "Z"=w256) -> (w253:T2)
        n96 = for {
          tunnel: w255 -> [w260]
          tunnel: T5[] [enum."    4.2 ¶b-Z²¾°Ê", enum."    4.3 ¶b-Z²¾°Êª¬ºA"] -> [w259] mode=indexing
          n97 = Enqueue Element(queue=w260, element=w259) -> ()  [unwired: 2 in, 3 out]
          n98 = Wait (ms)(milliseconds to wait=u32 2 ("millisecond multiple")) -> ()  [unwired: 1 out]
        }
      }
      frame "動作-Z移動-" {
        n99 = local read "單步距離(mm)"() -> (w263:dbl)
        n100 = Unbundle By Name(w269) -> ("Z"=w272:dbl)
        n101 = Add(x=w272, y=w263) -> (x+y=w271:dbl)
        n102 = Bundle By Name(cluster=w269, "Z"=w271) -> (w268:T2)
        n103 = for {
          tunnel: w270 -> [w275]
          tunnel: T5[] [enum."    4.2 ¶b-Z²¾°Ê", enum."    4.3 ¶b-Z²¾°Êª¬ºA"] -> [w274] mode=indexing
          n104 = Enqueue Element(queue=w275, element=w274) -> ()  [unwired: 2 in, 3 out]
          n105 = Wait (ms)(milliseconds to wait=u32 2 ("millisecond multiple")) -> ()  [unwired: 1 out]
        }
      }
      frame "動作-θ移動+" {
        n106 = local read "單步角度(degree)"() -> (w278:dbl)
        n107 = Unbundle By Name(w284) -> ("θ"=w287:dbl)
        n108 = Add(x=w287, y=w278) -> (x+y=w286:dbl)
        n109 = Bundle By Name(cluster=w284, "θ"=w286) -> (w283:T2)
        n110 = for {
          tunnel: w285 -> [w290]
          tunnel: T5[] [enum."    5.2 ¶b-£c²¾°Ê", enum."    5.3 ¶b-£c²¾°Êª¬ºA"] -> [w289] mode=indexing
          n111 = Enqueue Element(queue=w290, element=w289) -> ()  [unwired: 2 in, 3 out]
          n112 = Wait (ms)(milliseconds to wait=u32 2 ("millisecond multiple")) -> ()  [unwired: 1 out]
        }
      }
      frame "動作-θ移動-" {
        n113 = local read "單步角度(degree)"() -> (w293:dbl)
        n114 = Unbundle By Name(w299) -> ("θ"=w302:dbl)
        n115 = Subtract(x=w302, y=w293) -> (x-y=w301:dbl)
        n116 = Bundle By Name(cluster=w299, "θ"=w301) -> (w298:T2)
        n117 = for {
          tunnel: w300 -> [w305]
          tunnel: T5[] [enum."    5.2 ¶b-£c²¾°Ê", enum."    5.3 ¶b-£c²¾°Êª¬ºA"] -> [w304] mode=indexing
          n118 = Enqueue Element(queue=w305, element=w304) -> ()  [unwired: 2 in, 3 out]
          n119 = Wait (ms)(milliseconds to wait=u32 2 ("millisecond multiple")) -> ()  [unwired: 1 out]
        }
      }
      frame "1.0 ¶b-ªì©l¤Æ" {
        n120 = call "Main_Function_VISA.vi"("Delay Time"=u32 100, "Action_VISA"=T12."Open Connect", "VISA Data"=w324, "VISA In"=w330) -> ("Error Out"=w320:errorcluster, "VISA Out"=w307:refnum<visa-resource-name>)  [unwired: 5 in, 1 out]
        n121 = call "Main_Function_Motion Control.vi"("Motion_Action"=Control_Motion_Action."Servo On", "Error In"=w320, "Paremeter"=w328, "VISA In"=w307) -> ("Error Out"=w314:errorcluster, "VISA Out"=w311:refnum<visa-resource-name>)  [unwired: 5 in, 1 out]
        n122 = call "Main_Function_Motion Control.vi"("Motion_Action"=Control_Motion_Action."Servo On", "Error In"=w314, "Paremeter"=w327, "VISA In"=w311) -> ("Error Out"=w313:errorcluster, "VISA Out"=w310:refnum<visa-resource-name>)  [unwired: 5 in, 1 out]
        n123 = call "Main_Function_Motion Control.vi"("Motion_Action"=Control_Motion_Action."Servo On", "Error In"=w313, "Paremeter"=w326, "VISA In"=w310) -> ("Error Out"=w312:errorcluster, "VISA Out"=w309:refnum<visa-resource-name>)  [unwired: 5 in, 1 out]
        n124 = call "Main_Function_Motion Control.vi"("Motion_Action"=Control_Motion_Action."Servo On", "Error In"=w312, "Paremeter"=w325, "VISA In"=w309) -> ("Error Out"=w323:errorcluster)  [unwired: 5 in, 2 out]
      }
      frame "    1.1 ¶b-¶×¤J°Ñ¼Æ" {
        n125 = call "Main_Function_Motion Control.vi"("Motion_Action"=Control_Motion_Action."Set Speed", "Paremeter"=w334, "VISA In"=w335) -> ("Error Out"=w338:errorcluster, "VISA Out"=w343:refnum<visa-resource-name>)  [unwired: 6 in, 1 out]
        n126 = call "Main_Function_Motion Control.vi"("Motion_Action"=Control_Motion_Action."Set Acc", "Error In"=w338, "VISA In"=w343) -> ("Error Out"=w337:errorcluster, "VISA Out"=w339:refnum<visa-resource-name>)  [unwired: 6 in, 1 out]
        n127 = call "Main_Function_Motion Control.vi"("Motion_Action"=Control_Motion_Action."Set Deacc", "Error In"=w337, "VISA In"=w339) -> ("Error Out"=w336:errorcluster, "VISA Out"=w345:refnum<visa-resource-name>)  [unwired: 6 in, 1 out]
        n128 = call "Main_Function_Motion Control.vi"("Motion_Action"=Control_Motion_Action."Servo On", "Error In"=w336, "VISA In"=w345) -> ("Error Out"=w333:errorcluster)  [unwired: 6 in, 2 out]
      }
      frame "2.0 ¶b-X¦^­ìÂI" {
        n129 = call "Main_Function_Motion Control.vi"("Motion_Action"=Control_Motion_Action."Homing", "Paremeter"=w354, "VISA In"=w359) -> ("Error Out"=w353:errorcluster)  [unwired: 6 in, 2 out]
        n130 = call "Main_FGV_Time.vi"("Time Action"=enum16{"Start", "Read", "Clear"}."Start") -> ()  [unwired: 10 in, 1 out]
      }
      frame "    2.1 ¶b-Xª¬ºA" {
        n131 = call "Main_Function_Motion Control.vi"("Motion_Action"=Control_Motion_Action."Read Status", "Paremeter"=w366, "VISA In"=w371) -> ("Error Out"=w375:errorcluster, "Response"=w376:string)  [unwired: 6 in, 1 out]
        n132 = call "Main_SubVI_Hex to Result Array.vi"("Error In"=w375, "Hex In"=w376) -> ("Error Out"=w374:errorcluster, "Normal Array Out"=w378:string[])  [unwired: 8 in]
        n133 = call "Main_SubVI_Motion Status.vi"("Error In"=w374, "Normal Array In"=w378) -> ("Error Out"=w365:errorcluster, "Status"=w373:T14)  [unwired: 7 in, 1 out]
        n134 = case shown="Error" w365 {
          selector: w365 -> [_ w409]
          tunnel: w373 -> [w384 _]
          tunnel: w372 -> [w382 _]
          tunnel: w364 -> [w381 _]
          tunnel: [w380 Control_手動測試_手動測試_Action."2.0 ¶b-X¦^­ìÂI" ("手動測試-Action 2")] -> w363
          tunnel: [w379 w409] -> w362
          tunnel: w361 -> [_ _]
          frame No Error {
            n135 = Unbundle By Name(w384) -> ("Home_P"=w383:bool)
            n136 = case shown="False" w383 {
              tunnel: w382 -> [w391 w407]
              tunnel: w381 -> [w388 _]
              tunnel: [w386 Control_手動測試_手動測試_Action."9.0 等待" ("手動測試-Action 2")] -> w380
              tunnel: [w385 errorcluster {"status"=FALSE, "code"=0, "source"=""} ("Error Out")] -> w379
              frame False {
                n137 = call "Main_FGV_Time.vi"("Time Action"=enum16{"Start", "Read", "Clear"}."Read") -> ("Time"=w390:u32)  [unwired: 10 in]
                n138 = Greater Or Equal?(x=w390, y=w388) -> (x >= y?=w387:bool)
                n139 = case shown="False" w387 {
                  tunnel: w391 -> [w396 _]
                  tunnel: [Control_手動測試_手動測試_Action."9.0 等待" ("手動測試-Action 2") Control_手動測試_手動測試_Action."2.0 ¶b-X¦^­ìÂI" ("手動測試-Action 2")] -> w386
                  tunnel: [errorcluster {"status"=FALSE, "code"=0, "source"=""} ("Error Out") w399] -> w385
                  frame False {
                    n140 = Enqueue Element At Opposite End(queue=w396, element=Control_手動測試_手動測試_Action."    2.1 ¶b-Xª¬ºA" ("手動測試-Action")) -> (queue out=w397:refnum<queue>)  [unwired: 2 in, 2 out]
                    n141 = Enqueue Element At Opposite End(queue=w397, element=Control_手動測試_手動測試_Action."    2.4 ¶b-X¦ì¸m" ("手動測試-Action")) -> ()  [unwired: 2 in, 3 out]
                  }
                  frame True {
                    n142 = Bundle By Name(cluster=errorcluster {"status"=FALSE, "code"=0, "source"=""} ("Error Out"), "status"=TRUE, "source"="Error\nMove Timeout！") -> (w399:errorcluster)
                  }
                }
              }
              frame True {
                n143 = call "Main_FGV_Time.vi"("Time Action"=enum16{"Start", "Read", "Clear"}."Clear") -> ()  [unwired: 10 in, 1 out]
                n144 = Enqueue Element At Opposite End(queue=w407, element=Control_手動測試_手動測試_Action."    2.4 ¶b-X¦ì¸m" ("手動測試-Action")) -> ()  [unwired: 2 in, 3 out]
              }
            }
          }
          frame Error {
          }
        }
      }
      frame "    2.2 ¶b-X²¾°Ê" {
        n145 = Bundle By Name(cluster=w414, "Angle"=w419) -> (w427:T3)
        n146 = call "Main_Function_Motion Control.vi"("Motion_Action"=Control_Motion_Action."Set Position", "Paremeter"=w427, "VISA In"=w420) -> ("Error Out"=w426:errorcluster, "VISA Out"=w423:refnum<visa-resource-name>)  [unwired: 6 in, 1 out]
        n147 = call "Main_Function_Motion Control.vi"("Motion_Action"=Control_Motion_Action."Start Move", "Error In"=w426, "Paremeter"=w427, "VISA In"=w423) -> ("Error Out"=w425:errorcluster, "VISA Out"=w428:refnum<visa-resource-name>)  [unwired: 5 in, 1 out]
        n148 = call "Main_Function_Motion Control.vi"("Motion_Action"=Control_Motion_Action."Servo On", "Error In"=w425, "Paremeter"=w427, "VISA In"=w428) -> ("Error Out"=w413:errorcluster)  [unwired: 5 in, 2 out]
        n149 = call "Main_FGV_Time.vi"("Time Action"=enum16{"Start", "Read", "Clear"}."Start") -> ()  [unwired: 10 in, 1 out]
      }
      frame "    2.3 ¶b-X²¾°Êª¬ºA" {
        n150 = call "Main_Function_Motion Control.vi"("Motion_Action"=Control_Motion_Action."Read Status", "Paremeter"=w435, "VISA In"=w440) -> ("Error Out"=w442:errorcluster, "Response"=w443:string)  [unwired: 6 in, 1 out]
        n151 = call "Main_SubVI_Hex to Result Array.vi"("Error In"=w442, "Hex In"=w443) -> ("Error Out"=w441:errorcluster, "Normal Array Out"=w445:string[])  [unwired: 8 in]
        n152 = call "Main_SubVI_Motion Status.vi"("Error In"=w441, "Normal Array In"=w445) -> ("Error Out"=w430:errorcluster, "Status"=w433:T14)  [unwired: 7 in, 1 out]
        n153 = case shown="No Error" w430 {
          selector: w430 -> [_ w476]
          tunnel: w433 -> [w451 _]
          tunnel: w434 -> [w449 _]
          tunnel: w432 -> [w448 _]
          tunnel: [w447 Control_手動測試_手動測試_Action."    2.2 ¶b-X²¾°Ê" ("手動測試-Action 2")] -> w431
          tunnel: [w446 w476] -> w429
          frame No Error {
            n154 = Unbundle By Name(w451) -> ("Ready"=w450:bool)
            n155 = case shown="False" w450 {
              tunnel: w449 -> [w458 w474]
              tunnel: w448 -> [w455 _]
              tunnel: [w453 Control_手動測試_手動測試_Action."9.0 等待" ("手動測試-Action 2")] -> w447
              tunnel: [w452 errorcluster {"status"=FALSE, "code"=0, "source"=""} ("Error Out")] -> w446
              frame False {
                n156 = call "Main_FGV_Time.vi"("Time Action"=enum16{"Start", "Read", "Clear"}."Read") -> ("Time"=w457:u32)  [unwired: 10 in]
                n157 = Greater Or Equal?(x=w457, y=w455) -> (x >= y?=w454:bool)
                n158 = case shown="False" w454 {
                  tunnel: w458 -> [w463 _]
                  tunnel: [Control_手動測試_手動測試_Action."9.0 等待" ("手動測試-Action 2") Control_手動測試_手動測試_Action."    2.2 ¶b-X²¾°Ê" ("手動測試-Action 2")] -> w453
                  tunnel: [errorcluster {"status"=FALSE, "code"=0, "source"=""} ("Error Out") w466] -> w452
                  frame False {
                    n159 = Enqueue Element At Opposite End(queue=w463, element=Control_手動測試_手動測試_Action."    2.3 ¶b-X²¾°Êª¬ºA" ("手動測試-Action")) -> (queue out=w464:refnum<queue>)  [unwired: 2 in, 2 out]
                    n160 = Enqueue Element At Opposite End(queue=w464, element=Control_手動測試_手動測試_Action."    2.4 ¶b-X¦ì¸m" ("手動測試-Action")) -> ()  [unwired: 2 in, 3 out]
                  }
                  frame True {
                    n161 = Bundle By Name(cluster=errorcluster {"status"=FALSE, "code"=0, "source"=""} ("Error Out"), "status"=TRUE, "source"="Error\nMove Timeout！") -> (w466:errorcluster)
                  }
                }
              }
              frame True {
                n162 = call "Main_FGV_Time.vi"("Time Action"=enum16{"Start", "Read", "Clear"}."Clear") -> ()  [unwired: 10 in, 1 out]
                n163 = Enqueue Element At Opposite End(queue=w474, element=Control_手動測試_手動測試_Action."    2.4 ¶b-X¦ì¸m" ("手動測試-Action")) -> ()  [unwired: 2 in, 3 out]
              }
            }
          }
          frame Error {
          }
        }
      }
      frame "    2.4 ¶b-X¦ì¸m" {
        w495 = T4 1 items=["X"=1, "Y"=2, "Z"=3, "Rotation"=4] ("Axis Number")
        n164 = call "Main_Function_Motion Control.vi"("Motion_Action"=Control_Motion_Action."Read Position", "Paremeter"=w480, "VISA In"=w486) -> ("Error Out"=w490:errorcluster, "Response"=w491:string)  [unwired: 6 in, 1 out]
        n165 = call "Main_SubVI_Hex to Result Array.vi"("Error In"=w490, "Hex In"=w491) -> ("Error Out"=w492:errorcluster, "Normal Array Out"=w493:string[])  [unwired: 8 in]
        n166 = call "Main_SubVI_Motion Status.vi"("Error In"=w492, "Normal Array In"=w493) -> ("Error Out"=w489:errorcluster, "Response"=w488:string)  [unwired: 7 in, 1 out]
        n167 = call "Main_SubVI_Response to Pulse.vi"("Error In"=w489, "Response"=w488) -> ("Error Out"=w496:errorcluster, "Pulse"=w497:i32)  [unwired: 8 in]
        n168 = call "Main_SubVI_Pulse to Position.vi"("Error In"=w496, "Pulse"=w497, "Axis Number"=w495) -> ("Error Out"=w479:errorcluster, "Postion"=w494:dbl)  [unwired: 7 in]
        n169 = Bundle By Name(cluster=w485, "X軸位置(mm)"=w494) -> (w487:T1)
        n170 = local write "目前位置"(w487) -> ()
      }
      frame "    2.5 ¶b-X¶×¤J°Ñ¼Æ" {
        n171 = call "Main_Function_Motion Control.vi"("Motion_Action"=Control_Motion_Action."Set Speed", "Paremeter"=w505, "VISA In"=w506) -> ("Error Out"=w504:errorcluster, "VISA Out"=w511:refnum<visa-resource-name>)  [unwired: 6 in, 1 out]
        n172 = call "Main_Function_Motion Control.vi"("Motion_Action"=Control_Motion_Action."Set Acc", "Error In"=w504, "Paremeter"=w505, "VISA In"=w511) -> ("Error Out"=w503:errorcluster, "VISA Out"=w507:refnum<visa-resource-name>)  [unwired: 5 in, 1 out]
        n173 = call "Main_Function_Motion Control.vi"("Motion_Action"=Control_Motion_Action."Set Deacc", "Error In"=w503, "Paremeter"=w505, "VISA In"=w507) -> ("Error Out"=w502:errorcluster, "VISA Out"=w513:refnum<visa-resource-name>)  [unwired: 5 in, 1 out]
        n174 = call "Main_Function_Motion Control.vi"("Motion_Action"=Control_Motion_Action."Servo On", "Error In"=w502, "Paremeter"=w505, "VISA In"=w513) -> ("Error Out"=w501:errorcluster)  [unwired: 5 in, 2 out]
      }
      frame "3.0 ¶b-Y¦^­ìÂI" {
        n175 = call "Main_Function_Motion Control.vi"("Motion_Action"=Control_Motion_Action."Homing", "Paremeter"=w522, "VISA In"=w527) -> ("Error Out"=w521:errorcluster)  [unwired: 6 in, 2 out]
        n176 = call "Main_FGV_Time.vi"("Time Action"=enum16{"Start", "Read", "Clear"}."Start") -> ()  [unwired: 10 in, 1 out]
      }
      frame "    3.1 ¶b-Yª¬ºA" {
        n177 = call "Main_Function_Motion Control.vi"("Motion_Action"=Control_Motion_Action."Read Status", "Paremeter"=w536, "VISA In"=w541) -> ("Error Out"=w543:errorcluster, "Response"=w544:string)  [unwired: 6 in, 1 out]
        n178 = call "Main_SubVI_Hex to Result Array.vi"("Error In"=w543, "Hex In"=w544) -> ("Error Out"=w542:errorcluster, "Normal Array Out"=w546:string[])  [unwired: 8 in]
        n179 = call "Main_SubVI_Motion Status.vi"("Error In"=w542, "Normal Array In"=w546) -> ("Error Out"=w529:errorcluster, "Status"=w533:T14)  [unwired: 7 in, 1 out]
        n180 = case shown="Error" w529 {
          selector: w529 -> [_ w577]
          tunnel: w533 -> [w552 _]
          tunnel: w535 -> [w550 _]
          tunnel: w534 -> [w549 _]
          tunnel: [w548 Control_手動測試_手動測試_Action."3.0 ¶b-Y¦^­ìÂI" ("手動測試-Action 2")] -> w531
          tunnel: [w547 w577] -> w530
          tunnel: w532 -> [_ _]
          frame No Error {
            n181 = Unbundle By Name(w552) -> ("Home_P"=w551:bool)
            n182 = case shown="True" w551 {
              tunnel: w550 -> [w559 w575]
              tunnel: w549 -> [w556 _]
              tunnel: [w554 Control_手動測試_手動測試_Action."9.0 等待" ("手動測試-Action 2")] -> w548
              tunnel: [w553 errorcluster {"status"=FALSE, "code"=0, "source"=""} ("Error Out")] -> w547
              frame False {
                n183 = call "Main_FGV_Time.vi"("Time Action"=enum16{"Start", "Read", "Clear"}."Read") -> ("Time"=w558:u32)  [unwired: 10 in]
                n184 = Greater Or Equal?(x=w558, y=w556) -> (x >= y?=w555:bool)
                n185 = case shown="True" w555 {
                  tunnel: w559 -> [w564 _]
                  tunnel: [Control_手動測試_手動測試_Action."9.0 等待" ("手動測試-Action 2") Control_手動測試_手動測試_Action."3.0 ¶b-Y¦^­ìÂI" ("手動測試-Action 2")] -> w554
                  tunnel: [errorcluster {"status"=FALSE, "code"=0, "source"=""} ("Error Out") w567] -> w553
                  frame False {
                    n186 = Enqueue Element At Opposite End(queue=w564, element=Control_手動測試_手動測試_Action."    3.1 ¶b-Yª¬ºA" ("手動測試-Action")) -> (queue out=w565:refnum<queue>)  [unwired: 2 in, 2 out]
                    n187 = Enqueue Element At Opposite End(queue=w565, element=Control_手動測試_手動測試_Action."    3.4 ¶b-Y¦ì¸m" ("手動測試-Action")) -> ()  [unwired: 2 in, 3 out]
                  }
                  frame True {
                    n188 = Bundle By Name(cluster=errorcluster {"status"=FALSE, "code"=0, "source"=""} ("Error Out"), "status"=TRUE, "source"="Error\nMove Timeout！") -> (w567:errorcluster)
                  }
                }
              }
              frame True {
                n189 = call "Main_FGV_Time.vi"("Time Action"=enum16{"Start", "Read", "Clear"}."Clear") -> ()  [unwired: 10 in, 1 out]
                n190 = Enqueue Element At Opposite End(queue=w575, element=Control_手動測試_手動測試_Action."    3.4 ¶b-Y¦ì¸m" ("手動測試-Action")) -> ()  [unwired: 2 in, 3 out]
              }
            }
          }
          frame Error {
          }
        }
      }
      frame "    3.2 ¶b-Y²¾°Ê" {
        n191 = Bundle By Name(cluster=w582, "Angle"=w587) -> (w595:T3)
        n192 = call "Main_Function_Motion Control.vi"("Motion_Action"=Control_Motion_Action."Set Position", "Paremeter"=w595, "VISA In"=w588) -> ("Error Out"=w594:errorcluster, "VISA Out"=w591:refnum<visa-resource-name>)  [unwired: 6 in, 1 out]
        n193 = call "Main_Function_Motion Control.vi"("Motion_Action"=Control_Motion_Action."Start Move", "Error In"=w594, "Paremeter"=w595, "VISA In"=w591) -> ("Error Out"=w593:errorcluster, "VISA Out"=w596:refnum<visa-resource-name>)  [unwired: 5 in, 1 out]
        n194 = call "Main_Function_Motion Control.vi"("Motion_Action"=Control_Motion_Action."Servo On", "Error In"=w593, "Paremeter"=w595, "VISA In"=w596) -> ("Error Out"=w581:errorcluster)  [unwired: 5 in, 2 out]
        n195 = call "Main_FGV_Time.vi"("Time Action"=enum16{"Start", "Read", "Clear"}."Start") -> ()  [unwired: 10 in, 1 out]
      }
      frame "    3.3 ¶b-Y²¾°Êª¬ºA" {
        n196 = call "Main_Function_Motion Control.vi"("Motion_Action"=Control_Motion_Action."Read Status", "Paremeter"=w604, "VISA In"=w609) -> ("Error Out"=w611:errorcluster, "Response"=w612:string)  [unwired: 6 in, 1 out]
        n197 = call "Main_SubVI_Hex to Result Array.vi"("Error In"=w611, "Hex In"=w612) -> ("Error Out"=w610:errorcluster, "Normal Array Out"=w614:string[])  [unwired: 8 in]
        n198 = call "Main_SubVI_Motion Status.vi"("Error In"=w610, "Normal Array In"=w614) -> ("Error Out"=w603:errorcluster, "Status"=w597:T14)  [unwired: 7 in, 1 out]
        n199 = case shown="No Error" w603 {
          selector: w603 -> [_ w645]
          tunnel: w597 -> [w620 _]
          tunnel: w601 -> [w618 _]
          tunnel: w598 -> [w617 _]
          tunnel: [w616 Control_手動測試_手動測試_Action."    3.2 ¶b-Y²¾°Ê" ("手動測試-Action 2")] -> w599
          tunnel: [w615 w645] -> w602
          tunnel: w600 -> [_ _]
          frame No Error {
            n200 = Unbundle By Name(w620) -> ("Ready"=w619:bool)
            n201 = case shown="False" w619 {
              tunnel: w618 -> [w627 w643]
              tunnel: w617 -> [w624 _]
              tunnel: [w622 Control_手動測試_手動測試_Action."9.0 等待" ("手動測試-Action 2")] -> w616
              tunnel: [w621 errorcluster {"status"=FALSE, "code"=0, "source"=""} ("Error Out")] -> w615
              frame False {
                n202 = call "Main_FGV_Time.vi"("Time Action"=enum16{"Start", "Read", "Clear"}."Read") -> ("Time"=w626:u32)  [unwired: 10 in]
                n203 = Greater Or Equal?(x=w626, y=w624) -> (x >= y?=w623:bool)
                n204 = case shown="False" w623 {
                  tunnel: w627 -> [w632 _]
                  tunnel: [Control_手動測試_手動測試_Action."9.0 等待" ("手動測試-Action 2") Control_手動測試_手動測試_Action."    3.2 ¶b-Y²¾°Ê" ("手動測試-Action 2")] -> w622
                  tunnel: [errorcluster {"status"=FALSE, "code"=0, "source"=""} ("Error Out") w635] -> w621
                  frame False {
                    n205 = Enqueue Element At Opposite End(queue=w632, element=Control_手動測試_手動測試_Action."    3.3 ¶b-Y²¾°Êª¬ºA" ("手動測試-Action")) -> (queue out=w633:refnum<queue>)  [unwired: 2 in, 2 out]
                    n206 = Enqueue Element At Opposite End(queue=w633, element=Control_手動測試_手動測試_Action."    3.4 ¶b-Y¦ì¸m" ("手動測試-Action")) -> ()  [unwired: 2 in, 3 out]
                  }
                  frame True {
                    n207 = Bundle By Name(cluster=errorcluster {"status"=FALSE, "code"=0, "source"=""} ("Error Out"), "status"=TRUE, "source"="Error\nMove Timeout！") -> (w635:errorcluster)
                  }
                }
              }
              frame True {
                n208 = call "Main_FGV_Time.vi"("Time Action"=enum16{"Start", "Read", "Clear"}."Clear") -> ()  [unwired: 10 in, 1 out]
                n209 = Enqueue Element At Opposite End(queue=w643, element=Control_手動測試_手動測試_Action."    3.4 ¶b-Y¦ì¸m" ("手動測試-Action")) -> ()  [unwired: 2 in, 3 out]
              }
            }
          }
          frame Error {
          }
        }
      }
      frame "    3.4 ¶b-Y¦ì¸m" {
        w664 = T4 2 items=["X"=1, "Y"=2, "Z"=3, "Rotation"=4] ("Axis Number")
        n210 = call "Main_Function_Motion Control.vi"("Motion_Action"=Control_Motion_Action."Read Position", "Paremeter"=w649, "VISA In"=w656) -> ("Error Out"=w659:errorcluster, "Response"=w660:string)  [unwired: 6 in, 1 out]
        n211 = call "Main_SubVI_Hex to Result Array.vi"("Error In"=w659, "Hex In"=w660) -> ("Error Out"=w661:errorcluster, "Normal Array Out"=w662:string[])  [unwired: 8 in]
        n212 = call "Main_SubVI_Motion Status.vi"("Error In"=w661, "Normal Array In"=w662) -> ("Error Out"=w658:errorcluster, "Response"=w657:string)  [unwired: 7 in, 1 out]
        n213 = call "Main_SubVI_Response to Pulse.vi"("Error In"=w658, "Response"=w657) -> ("Error Out"=w665:errorcluster, "Pulse"=w666:i32)  [unwired: 8 in]
        n214 = call "Main_SubVI_Pulse to Position.vi"("Error In"=w665, "Pulse"=w666, "Axis Number"=w664) -> ("Error Out"=w648:errorcluster, "Postion"=w663:dbl)  [unwired: 7 in]
        n215 = Bundle By Name(cluster=w655, "Y軸位置(mm)"=w663) -> (w653:T1)
        n216 = local write "目前位置"(w653) -> ()
      }
      frame "    3.5 ¶b-Y¶×¤J°Ñ¼Æ" {
        n217 = call "Main_Function_Motion Control.vi"("Motion_Action"=Control_Motion_Action."Set Speed", "Paremeter"=w672, "VISA In"=w671) -> ("Error Out"=w679:errorcluster, "VISA Out"=w684:refnum<visa-resource-name>)  [unwired: 6 in, 1 out]
        n218 = call "Main_Function_Motion Control.vi"("Motion_Action"=Control_Motion_Action."Set Acc", "Error In"=w679, "Paremeter"=w672, "VISA In"=w684) -> ("Error Out"=w678:errorcluster, "VISA Out"=w680:refnum<visa-resource-name>)  [unwired: 5 in, 1 out]
        n219 = call "Main_Function_Motion Control.vi"("Motion_Action"=Control_Motion_Action."Set Deacc", "Error In"=w678, "Paremeter"=w672, "VISA In"=w680) -> ("Error Out"=w677:errorcluster, "VISA Out"=w686:refnum<visa-resource-name>)  [unwired: 5 in, 1 out]
        n220 = call "Main_Function_Motion Control.vi"("Motion_Action"=Control_Motion_Action."Servo On", "Error In"=w677, "Paremeter"=w672, "VISA In"=w686) -> ("Error Out"=w670:errorcluster)  [unwired: 5 in, 2 out]
      }
      frame "4.0 ¶b-Z¦^­ìÂI" {
        n221 = call "Main_Function_Motion Control.vi"("Motion_Action"=Control_Motion_Action."Homing", "Paremeter"=w691, "VISA In"=w696) -> ("Error Out"=w690:errorcluster)  [unwired: 6 in, 2 out]
        n222 = call "Main_FGV_Time.vi"("Time Action"=enum16{"Start", "Read", "Clear"}."Start") -> ()  [unwired: 10 in, 1 out]
      }
      frame "    4.1 ¶b-Zª¬ºA" {
        n223 = call "Main_Function_Motion Control.vi"("Motion_Action"=Control_Motion_Action."Read Status", "Paremeter"=w704, "VISA In"=w709) -> ("Error Out"=w711:errorcluster, "Response"=w712:string)  [unwired: 6 in, 1 out]
        n224 = call "Main_SubVI_Hex to Result Array.vi"("Error In"=w711, "Hex In"=w712) -> ("Error Out"=w710:errorcluster, "Normal Array Out"=w714:string[])  [unwired: 8 in]
        n225 = call "Main_SubVI_Motion Status.vi"("Error In"=w710, "Normal Array In"=w714) -> ("Error Out"=w703:errorcluster, "Status"=w699:T14)  [unwired: 7 in, 1 out]
        n226 = case shown="No Error" w703 {
          selector: w703 -> [_ w745]
          tunnel: w699 -> [w720 _]
          tunnel: w701 -> [w718 _]
          tunnel: w700 -> [w717 _]
          tunnel: [w716 Control_手動測試_手動測試_Action."4.0 ¶b-Z¦^­ìÂI" ("手動測試-Action 2")] -> w698
          tunnel: [w715 w745] -> w702
          frame No Error {
            n227 = Unbundle By Name(w720) -> ("Home_P"=w719:bool)
            n228 = case shown="True" w719 {
              tunnel: w718 -> [w727 w743]
              tunnel: w717 -> [w724 _]
              tunnel: [w722 Control_手動測試_手動測試_Action."9.0 等待" ("手動測試-Action 2")] -> w716
              tunnel: [w721 errorcluster {"status"=FALSE, "code"=0, "source"=""} ("Error Out")] -> w715
              frame False {
                n229 = call "Main_FGV_Time.vi"("Time Action"=enum16{"Start", "Read", "Clear"}."Read") -> ("Time"=w726:u32)  [unwired: 10 in]
                n230 = Greater Or Equal?(x=w726, y=w724) -> (x >= y?=w723:bool)
                n231 = case shown="False" w723 {
                  tunnel: w727 -> [w732 _]
                  tunnel: [Control_手動測試_手動測試_Action."9.0 等待" ("手動測試-Action 2") Control_手動測試_手動測試_Action."4.0 ¶b-Z¦^­ìÂI" ("手動測試-Action 2")] -> w722
                  tunnel: [errorcluster {"status"=FALSE, "code"=0, "source"=""} ("Error Out") w735] -> w721
                  frame False {
                    n232 = Enqueue Element At Opposite End(queue=w732, element=Control_手動測試_手動測試_Action."    4.1 ¶b-Zª¬ºA" ("手動測試-Action")) -> (queue out=w733:refnum<queue>)  [unwired: 2 in, 2 out]
                    n233 = Enqueue Element At Opposite End(queue=w733, element=Control_手動測試_手動測試_Action."    4.4 ¶b-Z¦ì¸m" ("手動測試-Action")) -> ()  [unwired: 2 in, 3 out]
                  }
                  frame True {
                    n234 = Bundle By Name(cluster=errorcluster {"status"=FALSE, "code"=0, "source"=""} ("Error Out"), "status"=TRUE, "source"="Error\nMove Timeout！") -> (w735:errorcluster)
                  }
                }
              }
              frame True {
                n235 = call "Main_FGV_Time.vi"("Time Action"=enum16{"Start", "Read", "Clear"}."Clear") -> ()  [unwired: 10 in, 1 out]
                n236 = Enqueue Element At Opposite End(queue=w743, element=Control_手動測試_手動測試_Action."    4.4 ¶b-Z¦ì¸m" ("手動測試-Action")) -> ()  [unwired: 2 in, 3 out]
              }
            }
          }
          frame Error {
          }
        }
      }
      frame "    4.2 ¶b-Z²¾°Ê" {
        n237 = Bundle By Name(cluster=w751, "Angle"=w755) -> (w763:T3)
        n238 = call "Main_Function_Motion Control.vi"("Motion_Action"=Control_Motion_Action."Set Position", "Paremeter"=w763, "VISA In"=w756) -> ("Error Out"=w762:errorcluster, "VISA Out"=w759:refnum<visa-resource-name>)  [unwired: 6 in, 1 out]
        n239 = call "Main_Function_Motion Control.vi"("Motion_Action"=Control_Motion_Action."Start Move", "Error In"=w762, "Paremeter"=w763, "VISA In"=w759) -> ("Error Out"=w761:errorcluster, "VISA Out"=w764:refnum<visa-resource-name>)  [unwired: 5 in, 1 out]
        n240 = call "Main_Function_Motion Control.vi"("Motion_Action"=Control_Motion_Action."Servo On", "Error In"=w761, "Paremeter"=w763, "VISA In"=w764) -> ("Error Out"=w749:errorcluster)  [unwired: 5 in, 2 out]
        n241 = call "Main_FGV_Time.vi"("Time Action"=enum16{"Start", "Read", "Clear"}."Start") -> ()  [unwired: 10 in, 1 out]
      }
      frame "    4.3 ¶b-Z²¾°Êª¬ºA" {
        n242 = call "Main_Function_Motion Control.vi"("Motion_Action"=Control_Motion_Action."Read Status", "Paremeter"=w771, "VISA In"=w776) -> ("Error Out"=w778:errorcluster, "Response"=w779:string)  [unwired: 6 in, 1 out]
        n243 = call "Main_SubVI_Hex to Result Array.vi"("Error In"=w778, "Hex In"=w779) -> ("Error Out"=w777:errorcluster, "Normal Array Out"=w781:string[])  [unwired: 8 in]
        n244 = call "Main_SubVI_Motion Status.vi"("Error In"=w777, "Normal Array In"=w781) -> ("Error Out"=w770:errorcluster, "Status"=w766:T14)  [unwired: 7 in, 1 out]
        n245 = case shown="No Error" w770 {
          selector: w770 -> [_ w812]
          tunnel: w766 -> [w787 _]
          tunnel: w767 -> [w785 _]
          tunnel: w765 -> [w784 _]
          tunnel: [w783 Control_手動測試_手動測試_Action."    4.2 ¶b-Z²¾°Ê" ("手動測試-Action 2")] -> w768
          tunnel: [w782 w812] -> w769
          frame No Error {
            n246 = Unbundle By Name(w787) -> ("Ready"=w786:bool)
            n247 = case shown="False" w786 {
              tunnel: w785 -> [w794 w810]
              tunnel: w784 -> [w791 _]
              tunnel: [w789 Control_手動測試_手動測試_Action."9.0 等待" ("手動測試-Action 2")] -> w783
              tunnel: [w788 errorcluster {"status"=FALSE, "code"=0, "source"=""} ("Error Out")] -> w782
              frame False {
                n248 = call "Main_FGV_Time.vi"("Time Action"=enum16{"Start", "Read", "Clear"}."Read") -> ("Time"=w793:u32)  [unwired: 10 in]
                n249 = Greater Or Equal?(x=w793, y=w791) -> (x >= y?=w790:bool)
                n250 = case shown="False" w790 {
                  tunnel: w794 -> [w799 _]
                  tunnel: [Control_手動測試_手動測試_Action."9.0 等待" ("手動測試-Action 2") Control_手動測試_手動測試_Action."    4.2 ¶b-Z²¾°Ê" ("手動測試-Action 2")] -> w789
                  tunnel: [errorcluster {"status"=FALSE, "code"=0, "source"=""} ("Error Out") w802] -> w788
                  frame False {
                    n251 = Enqueue Element At Opposite End(queue=w799, element=Control_手動測試_手動測試_Action."    4.3 ¶b-Z²¾°Êª¬ºA" ("手動測試-Action")) -> (queue out=w800:refnum<queue>)  [unwired: 2 in, 2 out]
                    n252 = Enqueue Element At Opposite End(queue=w800, element=Control_手動測試_手動測試_Action."    4.4 ¶b-Z¦ì¸m" ("手動測試-Action")) -> ()  [unwired: 2 in, 3 out]
                  }
                  frame True {
                    n253 = Bundle By Name(cluster=errorcluster {"status"=FALSE, "code"=0, "source"=""} ("Error Out"), "status"=TRUE, "source"="Error\nMove Timeout！") -> (w802:errorcluster)
                  }
                }
              }
              frame True {
                n254 = call "Main_FGV_Time.vi"("Time Action"=enum16{"Start", "Read", "Clear"}."Clear") -> ()  [unwired: 10 in, 1 out]
                n255 = Enqueue Element At Opposite End(queue=w810, element=Control_手動測試_手動測試_Action."    4.4 ¶b-Z¦ì¸m" ("手動測試-Action")) -> ()  [unwired: 2 in, 3 out]
              }
            }
          }
          frame Error {
          }
        }
      }
      frame "    4.4 ¶b-Z¦ì¸m" {
        w831 = T4 3 items=["X"=1, "Y"=2, "Z"=3, "Rotation"=4] ("Axis Number")
        n256 = call "Main_Function_Motion Control.vi"("Motion_Action"=Control_Motion_Action."Read Position", "Paremeter"=w816, "VISA In"=w822) -> ("Error Out"=w826:errorcluster, "Response"=w827:string)  [unwired: 6 in, 1 out]
        n257 = call "Main_SubVI_Hex to Result Array.vi"("Error In"=w826, "Hex In"=w827) -> ("Error Out"=w828:errorcluster, "Normal Array Out"=w829:string[])  [unwired: 8 in]
        n258 = call "Main_SubVI_Motion Status.vi"("Error In"=w828, "Normal Array In"=w829) -> ("Error Out"=w825:errorcluster, "Response"=w824:string)  [unwired: 7 in, 1 out]
        n259 = call "Main_SubVI_Response to Pulse.vi"("Error In"=w825, "Response"=w824) -> ("Error Out"=w832:errorcluster, "Pulse"=w833:i32)  [unwired: 8 in]
        n260 = call "Main_SubVI_Pulse to Position.vi"("Error In"=w832, "Pulse"=w833, "Axis Number"=w831) -> ("Error Out"=w815:errorcluster, "Postion"=w830:dbl)  [unwired: 7 in]
        n261 = Bundle By Name(cluster=w821, "Z軸位置(mm)"=w830) -> (w823:T1)
        n262 = local write "目前位置"(w823) -> ()
      }
      frame "    4.5 ¶b-Z¶×¤J°Ñ¼Æ" {
        n263 = call "Main_Function_Motion Control.vi"("Motion_Action"=Control_Motion_Action."Set Speed", "Paremeter"=w838, "VISA In"=w839) -> ("Error Out"=w842:errorcluster, "VISA Out"=w847:refnum<visa-resource-name>)  [unwired: 6 in, 1 out]
        n264 = call "Main_Function_Motion Control.vi"("Motion_Action"=Control_Motion_Action."Set Acc", "Error In"=w842, "Paremeter"=w838, "VISA In"=w847) -> ("Error Out"=w841:errorcluster, "VISA Out"=w843:refnum<visa-resource-name>)  [unwired: 5 in, 1 out]
        n265 = call "Main_Function_Motion Control.vi"("Motion_Action"=Control_Motion_Action."Set Deacc", "Error In"=w841, "Paremeter"=w838, "VISA In"=w843) -> ("Error Out"=w840:errorcluster, "VISA Out"=w849:refnum<visa-resource-name>)  [unwired: 5 in, 1 out]
        n266 = call "Main_Function_Motion Control.vi"("Motion_Action"=Control_Motion_Action."Servo On", "Error In"=w840, "Paremeter"=w838, "VISA In"=w849) -> ("Error Out"=w837:errorcluster)  [unwired: 5 in, 2 out]
      }
      frame "5.0 ¶b-£c¦^­ìÂI" {
        n267 = call "Main_Function_Motion Control.vi"("Motion_Action"=Control_Motion_Action."Homing", "Paremeter"=w858, "VISA In"=w863) -> ("Error Out"=w857:errorcluster)  [unwired: 6 in, 2 out]
        n268 = call "Main_FGV_Time.vi"("Time Action"=enum16{"Start", "Read", "Clear"}."Start") -> ()  [unwired: 10 in, 1 out]
      }
      frame "    5.1 ¶b-£cª¬ºA" {
        n269 = call "Main_Function_Motion Control.vi"("Motion_Action"=Control_Motion_Action."Read Status", "Paremeter"=w871, "VISA In"=w876) -> ("Error Out"=w878:errorcluster, "Response"=w879:string)  [unwired: 6 in, 1 out]
        n270 = call "Main_SubVI_Hex to Result Array.vi"("Error In"=w878, "Hex In"=w879) -> ("Error Out"=w877:errorcluster, "Normal Array Out"=w881:string[])  [unwired: 8 in]
        n271 = call "Main_SubVI_Motion Status.vi"("Error In"=w877, "Normal Array In"=w881) -> ("Error Out"=w870:errorcluster, "Status"=w869:T14)  [unwired: 7 in, 1 out]
        n272 = case shown="Error" w870 {
          selector: w870 -> [_ w913]
          tunnel: w869 -> [w887 _]
          tunnel: w866 -> [w885 _]
          tunnel: w865 -> [w884 _]
          tunnel: [w883 Control_手動測試_手動測試_Action."5.0 ¶b-£c¦^­ìÂI" ("手動測試-Action 2")] -> w867
          tunnel: [w882 w913] -> w868
          frame No Error {
            n273 = Unbundle By Name(w887) -> ("Home_P"=w886:bool)
            n274 = case shown="True" w886 {
              tunnel: w885 -> [w894 w911]
              tunnel: w884 -> [w891 _]
              tunnel: [w889 Control_手動測試_手動測試_Action."9.0 等待" ("手動測試-Action 2")] -> w883
              tunnel: [w888 errorcluster {"status"=FALSE, "code"=0, "source"=""} ("Error Out")] -> w882
              frame False {
                n275 = call "Main_FGV_Time.vi"("Time Action"=enum16{"Start", "Read", "Clear"}."Read") -> ("Time"=w893:u32)  [unwired: 10 in]
                n276 = Greater Or Equal?(x=w893, y=w891) -> (x >= y?=w890:bool)
                n277 = case shown="False" w890 {
                  tunnel: w894 -> [w899 _]
                  tunnel: [Control_手動測試_手動測試_Action."9.0 等待" ("手動測試-Action 2") Control_手動測試_手動測試_Action."5.0 ¶b-£c¦^­ìÂI" ("手動測試-Action 2")] -> w889
                  tunnel: [errorcluster {"status"=FALSE, "code"=0, "source"=""} ("Error Out") w903] -> w888
                  frame False {
                    n278 = Enqueue Element At Opposite End(queue=w899, element=Control_手動測試_手動測試_Action."    5.1 ¶b-£cª¬ºA" ("手動測試-Action")) -> (queue out=w900:refnum<queue>)  [unwired: 2 in, 2 out]
                    n279 = Enqueue Element At Opposite End(queue=w900, element=Control_手動測試_手動測試_Action."    5.4 ¶b-£c¦ì¸m" ("手動測試-Action")) -> ()  [unwired: 2 in, 3 out]
                  }
                  frame True {
                    n280 = Bundle By Name(cluster=errorcluster {"status"=FALSE, "code"=0, "source"=""} ("Error Out"), "status"=TRUE, "source"="Error\nMove Timeout！") -> (w903:errorcluster)
                    n281 = Wait (ms)(milliseconds to wait=u32 50) -> ()  [unwired: 1 out]
                  }
                }
              }
              frame True {
                n282 = call "Main_FGV_Time.vi"("Time Action"=enum16{"Start", "Read", "Clear"}."Clear") -> ()  [unwired: 10 in, 1 out]
                n283 = Enqueue Element At Opposite End(queue=w911, element=Control_手動測試_手動測試_Action."    5.4 ¶b-£c¦ì¸m" ("手動測試-Action")) -> ()  [unwired: 2 in, 3 out]
              }
            }
          }
          frame Error {
          }
        }
      }
      frame "    5.2 ¶b-£c²¾°Ê" {
        n284 = Bundle By Name(cluster=w918, "Angle"=w923) -> (w931:T3)
        n285 = call "Main_Function_Motion Control.vi"("Motion_Action"=Control_Motion_Action."Set Position", "Paremeter"=w931, "VISA In"=w924) -> ("Error Out"=w930:errorcluster, "VISA Out"=w927:refnum<visa-resource-name>)  [unwired: 6 in, 1 out]
        n286 = call "Main_Function_Motion Control.vi"("Motion_Action"=Control_Motion_Action."Start Move", "Error In"=w930, "Paremeter"=w931, "VISA In"=w927) -> ("Error Out"=w929:errorcluster, "VISA Out"=w932:refnum<visa-resource-name>)  [unwired: 5 in, 1 out]
        n287 = call "Main_Function_Motion Control.vi"("Motion_Action"=Control_Motion_Action."Servo On", "Error In"=w929, "Paremeter"=w931, "VISA In"=w932) -> ("Error Out"=w917:errorcluster)  [unwired: 5 in, 2 out]
        n288 = call "Main_FGV_Time.vi"("Time Action"=enum16{"Start", "Read", "Clear"}."Start") -> ()  [unwired: 10 in, 1 out]
      }
      frame "    5.3 ¶b-£c²¾°Êª¬ºA" {
        n289 = call "Main_Function_Motion Control.vi"("Motion_Action"=Control_Motion_Action."Read Status", "Paremeter"=w939, "VISA In"=w944) -> ("Error Out"=w946:errorcluster, "Response"=w947:string)  [unwired: 6 in, 1 out]
        n290 = call "Main_SubVI_Hex to Result Array.vi"("Error In"=w946, "Hex In"=w947) -> ("Error Out"=w945:errorcluster, "Normal Array Out"=w949:string[])  [unwired: 8 in]
        n291 = call "Main_SubVI_Motion Status.vi"("Error In"=w945, "Normal Array In"=w949) -> ("Error Out"=w938:errorcluster, "Status"=w933:T14)  [unwired: 7 in, 1 out]
        n292 = case shown="No Error" w938 {
          selector: w938 -> [_ w981]
          tunnel: w933 -> [w955 _]
          tunnel: w936 -> [w953 _]
          tunnel: w934 -> [w952 _]
          tunnel: [w951 Control_手動測試_手動測試_Action."    5.2 ¶b-£c²¾°Ê" ("手動測試-Action 2")] -> w935
          tunnel: [w950 w981] -> w937
          frame No Error {
            n293 = Unbundle By Name(w955) -> ("Ready"=w954:bool)
            n294 = case shown="True" w954 {
              tunnel: w953 -> [w962 w979]
              tunnel: w952 -> [w959 _]
              tunnel: [w957 Control_手動測試_手動測試_Action."9.0 等待" ("手動測試-Action 2")] -> w951
              tunnel: [w956 errorcluster {"status"=FALSE, "code"=0, "source"=""} ("Error Out")] -> w950
              frame False {
                n295 = call "Main_FGV_Time.vi"("Time Action"=enum16{"Start", "Read", "Clear"}."Read") -> ("Time"=w961:u32)  [unwired: 10 in]
                n296 = Greater Or Equal?(x=w961, y=w959) -> (x >= y?=w958:bool)
                n297 = case shown="True" w958 {
                  tunnel: w962 -> [w968 _]
                  tunnel: [Control_手動測試_手動測試_Action."9.0 等待" ("手動測試-Action 2") Control_手動測試_手動測試_Action."    5.2 ¶b-£c²¾°Ê" ("手動測試-Action 2")] -> w957
                  tunnel: [errorcluster {"status"=FALSE, "code"=0, "source"=""} ("Error Out") w971] -> w956
                  frame False {
                    n298 = Wait (ms)(milliseconds to wait=u32 50) -> ()  [unwired: 1 out]
                    n299 = Enqueue Element At Opposite End(queue=w968, element=Control_手動測試_手動測試_Action."    5.3 ¶b-£c²¾°Êª¬ºA" ("手動測試-Action")) -> (queue out=w969:refnum<queue>)  [unwired: 2 in, 2 out]
                    n300 = Enqueue Element At Opposite End(queue=w969, element=Control_手動測試_手動測試_Action."    5.4 ¶b-£c¦ì¸m" ("手動測試-Action")) -> ()  [unwired: 2 in, 3 out]
                  }
                  frame True {
                    n301 = Bundle By Name(cluster=errorcluster {"status"=FALSE, "code"=0, "source"=""} ("Error Out"), "status"=TRUE, "source"="Error\nMove Timeout！") -> (w971:errorcluster)
                  }
                }
              }
              frame True {
                n302 = call "Main_FGV_Time.vi"("Time Action"=enum16{"Start", "Read", "Clear"}."Clear") -> ()  [unwired: 10 in, 1 out]
                n303 = Enqueue Element At Opposite End(queue=w979, element=Control_手動測試_手動測試_Action."    5.4 ¶b-£c¦ì¸m" ("手動測試-Action")) -> ()  [unwired: 2 in, 3 out]
              }
            }
          }
          frame Error {
          }
        }
      }
      frame "    5.4 ¶b-£c¦ì¸m" {
        w1000 = T4 4 items=["X"=1, "Y"=2, "Z"=3, "Rotation"=4] ("Axis Number")
        n304 = call "Main_Function_Motion Control.vi"("Motion_Action"=Control_Motion_Action."Read Position", "Paremeter"=w985, "VISA In"=w991) -> ("Error Out"=w995:errorcluster, "Response"=w996:string)  [unwired: 6 in, 1 out]
        n305 = call "Main_SubVI_Hex to Result Array.vi"("Error In"=w995, "Hex In"=w996) -> ("Error Out"=w997:errorcluster, "Normal Array Out"=w998:string[])  [unwired: 8 in]
        n306 = call "Main_SubVI_Motion Status.vi"("Error In"=w997, "Normal Array In"=w998) -> ("Error Out"=w994:errorcluster, "Response"=w993:string)  [unwired: 7 in, 1 out]
        n307 = call "Main_SubVI_Response to Pulse.vi"("Error In"=w994, "Response"=w993) -> ("Error Out"=w1001:errorcluster, "Pulse"=w1002:i32)  [unwired: 8 in]
        n308 = call "Main_SubVI_Pulse to Position.vi"("Error In"=w1001, "Pulse"=w1002, "Axis Number"=w1000) -> ("Error Out"=w984:errorcluster, "Postion"=w999:dbl)  [unwired: 7 in]
        n309 = Bundle By Name(cluster=w990, "θ軸位置(degree)"=w999) -> (w992:T1)
        n310 = local write "目前位置"(w992) -> ()
      }
      frame "    5.5 ¶b-£c¶×¤J°Ñ¼Æ" {
        n311 = call "Main_Function_Motion Control.vi"("Motion_Action"=Control_Motion_Action."Set Speed", "Paremeter"=w1007, "VISA In"=w1008) -> ("Error Out"=w1011:errorcluster, "VISA Out"=w1016:refnum<visa-resource-name>)  [unwired: 6 in, 1 out]
        n312 = call "Main_Function_Motion Control.vi"("Motion_Action"=Control_Motion_Action."Set Acc", "Error In"=w1011, "Paremeter"=w1007, "VISA In"=w1016) -> ("Error Out"=w1010:errorcluster, "VISA Out"=w1012:refnum<visa-resource-name>)  [unwired: 5 in, 1 out]
        n313 = call "Main_Function_Motion Control.vi"("Motion_Action"=Control_Motion_Action."Set Deacc", "Error In"=w1010, "Paremeter"=w1007, "VISA In"=w1012) -> ("Error Out"=w1009:errorcluster, "VISA Out"=w1018:refnum<visa-resource-name>)  [unwired: 5 in, 1 out]
        n314 = call "Main_Function_Motion Control.vi"("Motion_Action"=Control_Motion_Action."Servo On", "Error In"=w1009, "Paremeter"=w1007, "VISA In"=w1018) -> ("Error Out"=w1006:errorcluster)  [unwired: 5 in, 2 out]
      }
      frame "6.0 ¶b-µ¥«Ý" {
        n315 = call "Main_Function_Motion Control.vi"("Motion_Action"=Control_Motion_Action."Servo On", "Paremeter"=w1026, "VISA In"=w1031) -> ("Error Out"=w1025:errorcluster)  [unwired: 6 in, 2 out]
      }
      frame "7.0 ¶b-µ²§ô" {
        n316 = call "Main_Function_Motion Control.vi"("Motion_Action"=Control_Motion_Action."Servo Off", "Paremeter"=w1040, "VISA In"=w1043) -> ("Error Out"=w1048:errorcluster, "VISA Out"=w1051:refnum<visa-resource-name>)  [unwired: 6 in, 1 out]
        n317 = call "Main_Function_Motion Control.vi"("Motion_Action"=Control_Motion_Action."Servo Off", "Error In"=w1048, "Paremeter"=w1039, "VISA In"=w1051) -> ("Error Out"=w1049:errorcluster, "VISA Out"=w1052:refnum<visa-resource-name>)  [unwired: 5 in, 1 out]
        n318 = call "Main_Function_Motion Control.vi"("Motion_Action"=Control_Motion_Action."Servo Off", "Error In"=w1049, "Paremeter"=w1038, "VISA In"=w1052) -> ("Error Out"=w1050:errorcluster, "VISA Out"=w1053:refnum<visa-resource-name>)  [unwired: 5 in, 1 out]
        n319 = call "Main_Function_Motion Control.vi"("Motion_Action"=Control_Motion_Action."Servo Off", "Error In"=w1050, "Paremeter"=w1037, "VISA In"=w1053) -> ("Error Out"=w1056:errorcluster, "VISA Out"=w1055:refnum<visa-resource-name>)  [unwired: 5 in, 1 out]
        n320 = call "Main_Function_VISA.vi"("Delay Time"=u32 50, "Action_VISA"=T12."Close Connect", "Error In"=w1056, "VISA Data"=w1041, "VISA In"=w1055) -> ("Error Out"=w1035:errorcluster)  [unwired: 4 in, 2 out]
        n321 = call <vilib>:"Clear Errors.vi"("error in (no error)"=w1035) -> ("error out"=w1034:errorcluster)  [unwired: 5 in, 1 out]
      }
      frame "8.0 量測" {
      }
      frame "    8.1 量測-初始化" {
        n322 = call "Measure_FUN_VISA.vi"("VISA Action"=Control_Measure_VISA_action."1.0 Initialize", "VISA Paremeter"=T13 {"Baud rate"=19200, "Data bits"=8, "Parity"=enum."None", "Stop bits"=10, "Flow control"=0}, "VISA In"=refnum<visa-resource-name> "COM9") -> ("Error Out"=w1070:errorcluster, "VISA Out"=w1079:refnum<visa-resource-name>)  [unwired: 6 in, 1 out]
        n323 = call "Measure_FUN_VISA.vi"("VISA Action"=Control_Measure_VISA_action."2.0 Power ON", "Error In"=w1070, "VISA In"=w1079) -> ("Error Out"=w1069:errorcluster, "VISA Out"=w1071:refnum<visa-resource-name>)  [unwired: 6 in, 1 out]
        n324 = call "Measure_FUN_VISA.vi"("VISA Action"=Control_Measure_VISA_action."2.5.2 DC*10 Mode", "Error In"=w1069, "VISA In"=w1071) -> ("Error Out"=w1068:errorcluster, "VISA Out"=w1074:refnum<visa-resource-name>)  [unwired: 6 in, 1 out]
        n325 = call "Measure_FUN_Read value.vi"("Read Action"=enum16{"Initialize", "Read Value", "Read State"}."Read State", "Error In"=w1068, "VISA In"=w1074) -> ("Error Out"=w1067:errorcluster)  [unwired: 5 in, 3 out]
      }
      frame "    8.2 量測-量測" {
      }
      frame "    8.2 量測-顯示結果" {
      }
      frame "    8.3 量測-離開" {
      }
      frame "9.0 等待" {
      }
      frame "10.0 離開" {
      }
      frame "    10.1 離開程式" {
        n326 = property on="確認離開" class="Bool (strict)"("Val(Sgnl)"=TRUE ("Value (Signaling)")) -> ()  [unwired: 2 in, 2 out]
      }
      frame "11.0 錯誤" {
      }
      frame "    11.1 錯誤-顯示錯誤" {
        n327 = Flush Queue(queue=w1143) -> (queue out=w1142:refnum<queue>)  [unwired: 1 in, 2 out]
      }
      frame "    11.2 錯誤-急停" {
        n328 = Flush Queue(queue=w1151) -> (queue out=w1150:refnum<queue>)  [unwired: 1 in, 2 out]
      }
    }
    n329 = case shown="Error" w98 {
      selector: w98 -> [_ w122]
      tunnel: w97 -> [_ w121]
      tunnel: w96 -> [_ w120]
      frame No Error {
      }
      frame Error {
        n330 = stacked-sequence {
          seq-local: [w123 _] -> [_ w130]
          tunnel: w121 -> [w124 _]
          tunnel: w122 -> [w127 _]
          tunnel: w120 -> [_ w131]
          frame #0 {
            n331 = Unbundle By Name(w127) -> ("source"=w126:string)
            n332 = call "6.Bounce Window_ERROR.vi"("MSG In"=w126) -> ("Error Action Out"=w125:T15)  [unwired: 10 in]
            n333 = case shown="\"Stop\"" w125 {
              tunnel: w124 -> [w128 _]
              tunnel: [w128 Control_手動測試_手動測試_Action."    11.1 錯誤-顯示錯誤" ("手動測試-Action")] -> w123
              frame "Try Again", Default {
              }
              frame "Stop" {
              }
            }
          }
          frame #1 {
            n334 = Enqueue Element At Opposite End(queue=w131, element=w130) -> ()  [unwired: 2 in, 3 out]
          }
        }
      }
    }
  }
  n335 = while {
    tunnel: [w1155] -> w9
    tunnel: [w1156] -> w8
    tunnel: w7 -> [w1162]
    tunnel: w5 -> [w1161]
    tunnel: w6 -> [w1160]
    stop <- w1152 stop-if-true
    n336 = VISA Wait on Event(7:u32 500 ("timeout (0)"), 8:w1160, 10:w1161, 11:w1162) -> (0:w1154:errorcluster, 3:w1158:refnum<visa-resource-name>)  [unwired: 1 in, 2 out]
    n337 = call "Measure_FUN_Read value.vi"("Read Action"=enum16{"Initialize", "Read Value", "Read State"}."Read Value", "Error In"=w1154, "VISA In"=w1158) -> ("Error Out"=w1155:errorcluster, "Value"=→"量測值(T)":dbl, "VISA Out"=w1156:refnum<visa-resource-name>)  [unwired: 5 in, 1 out]
    n338 = property on="確認離開" class="Bool (strict)"() -> ("Value"=w1152:bool)  [unwired: 2 in, 2 out]
  }
  n339 = VISA Flush I/O Buffer(VISA resource name=w8, error in (no error)=w9) -> (VISA resource name out=w3:refnum<visa-resource-name>, error out=w2:errorcluster)  [unwired: 1 in]
  n340 = call "Measure_FUN_VISA.vi"("VISA Action"=Control_Measure_VISA_action."5.0 Close", "Error In"=w2, "VISA In"=w3) -> ("Error Out"=w1:errorcluster)  [unwired: 6 in, 2 out]
  n341 = call <vilib>:"Clear Errors.vi"("error in (no error)"=w1) -> ()  [unwired: 5 in, 2 out]
